vi "CTRE_Phoenix_MotorControl_GetAllConfigSettingsEnhanced.vi"(6 "timeoutMs":i32=50, 8 "error in (no error)":errorcluster, 11 "PhoenixMotorControlDevRef":T12={"DeviceStatus"={"status"=FALSE, "code"=0, "source"=""}, "Type"=enum."PWM", "PWM"={"PWM Channel"=enum."PWM 1", "DeadBand"={"Name"="", "maxPositivePwm"=0, "minPositivePwm"=0, "centerPwm"=0, "maxNegativePwm"=0, "minNegativePwm"=0, "angularRange"=0}}, "CAN"={"Device Number"=0, "SetOutput VI Ref"=variant(enum8{"Percent VBus", "Current", "Speed", "Position", "Voltage"} enum."Percent VBus"), "GetOutput VI Ref"=variant(refnum<k1> refnum), "Enable VI Ref"=variant(dbl 12.0), "Disable VI Ref"=variant(enum8{"Percent VBus", "Speed", "Position", "Slave", "Unchanged / Invalid", "Voltage Compensation", "Current", "Motion Profile"} enum."Percent VBus"), "Data"=variant}, "Invert"=FALSE, "DIO PWM"={"PWM \"Enable\" Channel"=enum."Invalid", "DIOChannel"=enum."Invalid", "PWM Rate"=0.0}}) -> (0 "error out":errorcluster, 2 "Enhanced Motor Controller Configurables":T1={"Base Configurables"={"openLoopRamp"=0.0, "closedLoopRamp"=0.0, "peakOutputForward"=1.0, "peakOutputReverse"=-1.0, "nominalOutputForward"=0.0, "nominalOutputReverse"=0.0, "neutralDeadband"=0.04, "voltageCompSaturation"=0.0, "voltageMeasurementFilter"=32, "velocityMeasurementPeriod"=100, "velocityMeasurementWindow"=64, "forwardSoftLimitThreshold"=64, "reverseSoftLimitThreshold"=64, "forwardSoftLimitEnable"=FALSE, "reverseSoftLimitEnable"=FALSE, "slot0"={"P"=0.0, "I"=0.0, "D"=0.0, "F"=0.0, "integralZone"=0.0, "allowableClosedLoopError"=0, "maxIntegralAccumulator"=0.0, "closedLoopPeakOutput"=1.0, "closedLoopPeriod"=1}, "slot1"={"P"=0.0, "I"=0.0, "D"=0.0, "F"=0.0, "integralZone"=0.0, "allowableClosedLoopError"=0, "maxIntegralAccumulator"=0.0, "closedLoopPeakOutput"=1.0, "closedLoopPeriod"=1}, "slot2"={"P"=0.0, "I"=0.0, "D"=0.0, "F"=0.0, "integralZone"=0.0, "allowableClosedLoopError"=0, "maxIntegralAccumulator"=0.0, "closedLoopPeakOutput"=1.0, "closedLoopPeriod"=1}, "slot3"={"P"=0.0, "I"=0.0, "D"=0.0, "F"=0.0, "integralZone"=0.0, "allowableClosedLoopError"=0, "maxIntegralAccumulator"=0.0, "closedLoopPeakOutput"=1.0, "closedLoopPeriod"=1}, "auxPIDPolarity"=FALSE, "remoteFilter0"={"remoteSensorDeviceID"=0, "remoteSensorSource"=enum."Off"}, "remoteFilter1"={"remoteSensorDeviceID"=0, "remoteSensorSource"=enum."Off"}, "motionCruiseVelocity"=0, "motionAcceleration"=0, "motionProfileTrajectoryPeriod"=0, "feedbackNotContinuous"=FALSE, "remoteSensorClosedLoopDisableNeutralOnLOS"=FALSE, "clearPositionOnLimitF"=FALSE, "clearPositionOnLimitR"=FALSE, "clearPositionOnQuadIdx"=FALSE, "limitSwitchDisableNeutralOnLOS"=FALSE, "softLimitDisableNeutralOnLOS"=FALSE, "pulseWidthPeriod_EdgesPerRot"=1, "pulseWidthPeriod_FilterWindowSz"=1, "customParam"={"customParam0"=0, "customParam1"=0}, "trajectoryInterpolationEnable"=TRUE}, "primaryPID"={"selectedFeedbackCoefficient"=1.0, "selectedFeedbackSensor"=0}, "auxiliaryPID"={"selectedFeedbackCoefficient"=1.0, "selectedFeedbackSensor"=0}, "sum0Term"=0, "sum1Term"=0, "diff0Term"=0, "diff1Term"=0, "forwardLimitSwitchNormal"=enum."Normally Open", "reverseLimitSwitchNormal"=enum."Normally Open", "forwardLimitSwitchDeviceID"=0, "reverseLimitSwitchDeviceID"=0, "forwardLimitSwitchSource"=enum."Feedback Connector", "reverseLimitSwitchSource"=enum."Feedback Connector", "peakCurrentLimit"=1, "peakCurrentDuration"=1, "continuousCurrentLimit"=1} {"diff1Term" items=["QuadEncoder"=0, "Analog"=2, "Tachometer"=4, "Pulse Width Encoded Position"=8, "Remote Source 0"=11, "Remote Source 1"=12, "Software Emulated"=15]; "diff0Term" items=["QuadEncoder"=0, "Analog"=2, "Tachometer"=4, "Pulse Width Encoded Position"=8, "Remote Source 0"=11, "Remote Source 1"=12, "Software Emulated"=15]; "sum1Term" items=["QuadEncoder"=0, "Analog"=2, "Tachometer"=4, "Pulse Width Encoded Position"=8, "Remote Source 0"=11, "Remote Source 1"=12, "Software Emulated"=15]; "sum0Term" items=["QuadEncoder"=0, "Analog"=2, "Tachometer"=4, "Pulse Width Encoded Position"=8, "Remote Source 0"=11, "Remote Source 1"=12, "Software Emulated"=15]; "auxiliaryPID"."selectedFeedbackSensor" items=["QuadEncoder"=0, "Analog"=2, "Tachometer"=4, "Pulse Width Encoded Position"=8, "Sensor Sum (S0 + S1)"=9, "Sensor Difference (D0 - D1)"=10, "Remote Source 0"=11, "Remote Source 1"=12, "Software Emulated"=15]; "primaryPID"."selectedFeedbackSensor" items=["QuadEncoder"=0, "Analog"=2, "Tachometer"=4, "Pulse Width Encoded Position"=8, "Sensor Sum (S0 + S1)"=9, "Sensor Difference (D0 - D1)"=10, "Remote Source 0"=11, "Remote Source 1"=12, "Software Emulated"=15]; "Base Configurables"."velocityMeasurementPeriod" items=["Period_1ms"=1, "Period_2ms"=2, "Period_5ms"=5, "Period_10ms"=10, "Period_20ms"=20, "Period_25ms"=25, "Period_50ms"=50, "Period_100ms"=100]}, 3 "PhoenixMotorControlDevRef":T12={"DeviceStatus"={"status"=FALSE, "code"=0, "source"=""}, "Type"=enum."PWM", "PWM"={"PWM Channel"=enum."PWM 1", "DeadBand"={"Name"="", "maxPositivePwm"=0, "minPositivePwm"=0, "centerPwm"=0, "maxNegativePwm"=0, "minNegativePwm"=0, "angularRange"=0}}, "CAN"={"Device Number"=0, "SetOutput VI Ref"=variant(enum8{"Percent VBus", "Current", "Speed", "Position", "Voltage"} enum."Percent VBus"), "GetOutput VI Ref"=variant(refnum<k1> refnum), "Enable VI Ref"=variant(dbl 12.0), "Disable VI Ref"=variant(enum8{"Percent VBus", "Speed", "Position", "Slave", "Unchanged / Invalid", "Voltage Compensation", "Current", "Motion Profile"} enum."Percent VBus"), "Data"=variant}, "Invert"=FALSE, "DIO PWM"={"PWM \"Enable\" Channel"=enum."Invalid", "DIOChannel"=enum."Invalid", "PWM Rate"=0.0}})   [LabVIEW 2020]
doc: "Gets all the slot persistant settings"
uses:
  <vilib>/Rock Robotics/WPI/MotorControl/WPI_MotorControlDeviceRef.ctl
  <vilib>/Rock Robotics/WPI/MotorControl/WPI_MotorControlType.ctl
  <vilib>/Rock Robotics/SystemInterfaces/DIO/FPGA_DIOPWMChannel.ctl
  <vilib>/Rock Robotics/WPI/PWM/WPI_PWMDeadband.ctl
  <vilib>/Rock Robotics/SystemInterfaces/DIO/FPGA_DIOChannel.ctl
  <vilib>/Rock Robotics/WPI/ThirdParty/Phoenix-LabVIEW/Motor Controller/Controls/CTRE_Phoenix_MotorControl_EnhancedMotorControllerConfigurables.ctl
  <vilib>/Rock Robotics/WPI/ThirdParty/Phoenix-LabVIEW/Motor Controller/Controls/CTRE_Phoenix_MotorControl_BaseConfigurables.ctl
  <vilib>/Rock Robotics/WPI/ThirdParty/Phoenix-LabVIEW/Motor Controller/Controls/CTRE_Phoenix_MotorControl_VelocityMeasurementPeriod.ctl
  <vilib>/Rock Robotics/WPI/ThirdParty/Phoenix-LabVIEW/Motor Controller/Controls/CTRE_Phoenix_MotorControl_SlotStructure.ctl
  <vilib>/Rock Robotics/WPI/ThirdParty/Phoenix-LabVIEW/Motor Controller/Controls/CTRE_Phoenix_MotorControl_FilterStruct.ctl
  <vilib>/Rock Robotics/WPI/ThirdParty/Phoenix-LabVIEW/Motor Controller/Controls/CTRE_Phoenix_MotorControl_RemoteSourceType.ctl
  <vilib>/Rock Robotics/WPI/ThirdParty/Phoenix-LabVIEW/Controls/CTRE_Phoenix_CustomParamConfiguration.ctl
  <vilib>/Rock Robotics/WPI/ThirdParty/Phoenix-LabVIEW/Motor Controller/Controls/CTRE_Phoenix_MotorControl_FeedbackDevice.ctl
  <vilib>/Rock Robotics/WPI/ThirdParty/Phoenix-LabVIEW/Motor Controller/Controls/CTRE_Phoenix_MotorControl_SensorTermFeedbackDevice_Enhanced.ctl
  <vilib>/Rock Robotics/WPI/ThirdParty/Phoenix-LabVIEW/Motor Controller/Controls/CTRE_Phoenix_MotorControl_LimitSwitchNormal.ctl
  <vilib>/Rock Robotics/WPI/ThirdParty/Phoenix-LabVIEW/Motor Controller/Controls/CTRE_Phoenix_MotorControl_LimitSwitchSource_Local.ctl
  <vilib>/Rock Robotics/WPI/ThirdParty/Phoenix-LabVIEW/Controls/CTRE_Phoenix_Params.ctl
panel:
  # "Sum and Diff terms are ways to select more than one sensor as a feedback device. \n Sum 0 is the first feedback device to be used for the Sum term.\n Sum 1 is the feedback device to be added to Sum 0 for the Sum term.\n Diff 0 and Diff 1 work in a similar manner."
  # "These are only applicable\nif using a remote limit switch.\n\nLocal limit switches/no limit\nswitches do not use this."
  # "Current is below Continuous threshold AND\n\n(Requested output is weaker** than applied motor\noutput OR is in the opposite direction).\n/\nMotor output is set to requested output."
  # "Current is above Peak* Threshold for Peak Duration.\n/\nReduce motor output (towards neutral)."
  # "Current is below Continuous threshold.\n/\nRamp motor output towards requested output."
  # "Current is above Continuous threshold.\n/\nReduce motor output (towards neutral)."
  # "Current Limiting is NOT enabled\nby default.\nCall this VI to enable."
  # "*If the configured Peak Threshold is less than the Continuous Threshold, the applied Peak Threshold is set equal to the Configured Continuous Threshold in firmware.\n** Both requested output and applied motor output are in the same direction, and requested output is closer to neutral."
  # "False: Primary Output = PID[0] + PID[1]  ---  Auxiliary Output = PID[0] - PID[1]\nTrue:  Primary Output = PID[0] - PID[1] --- Auxiliary Output = PID[0] + PID[1]"
  # "Enable the motion profile executor to perform linear interpolation between profile points.  Defaults to True."
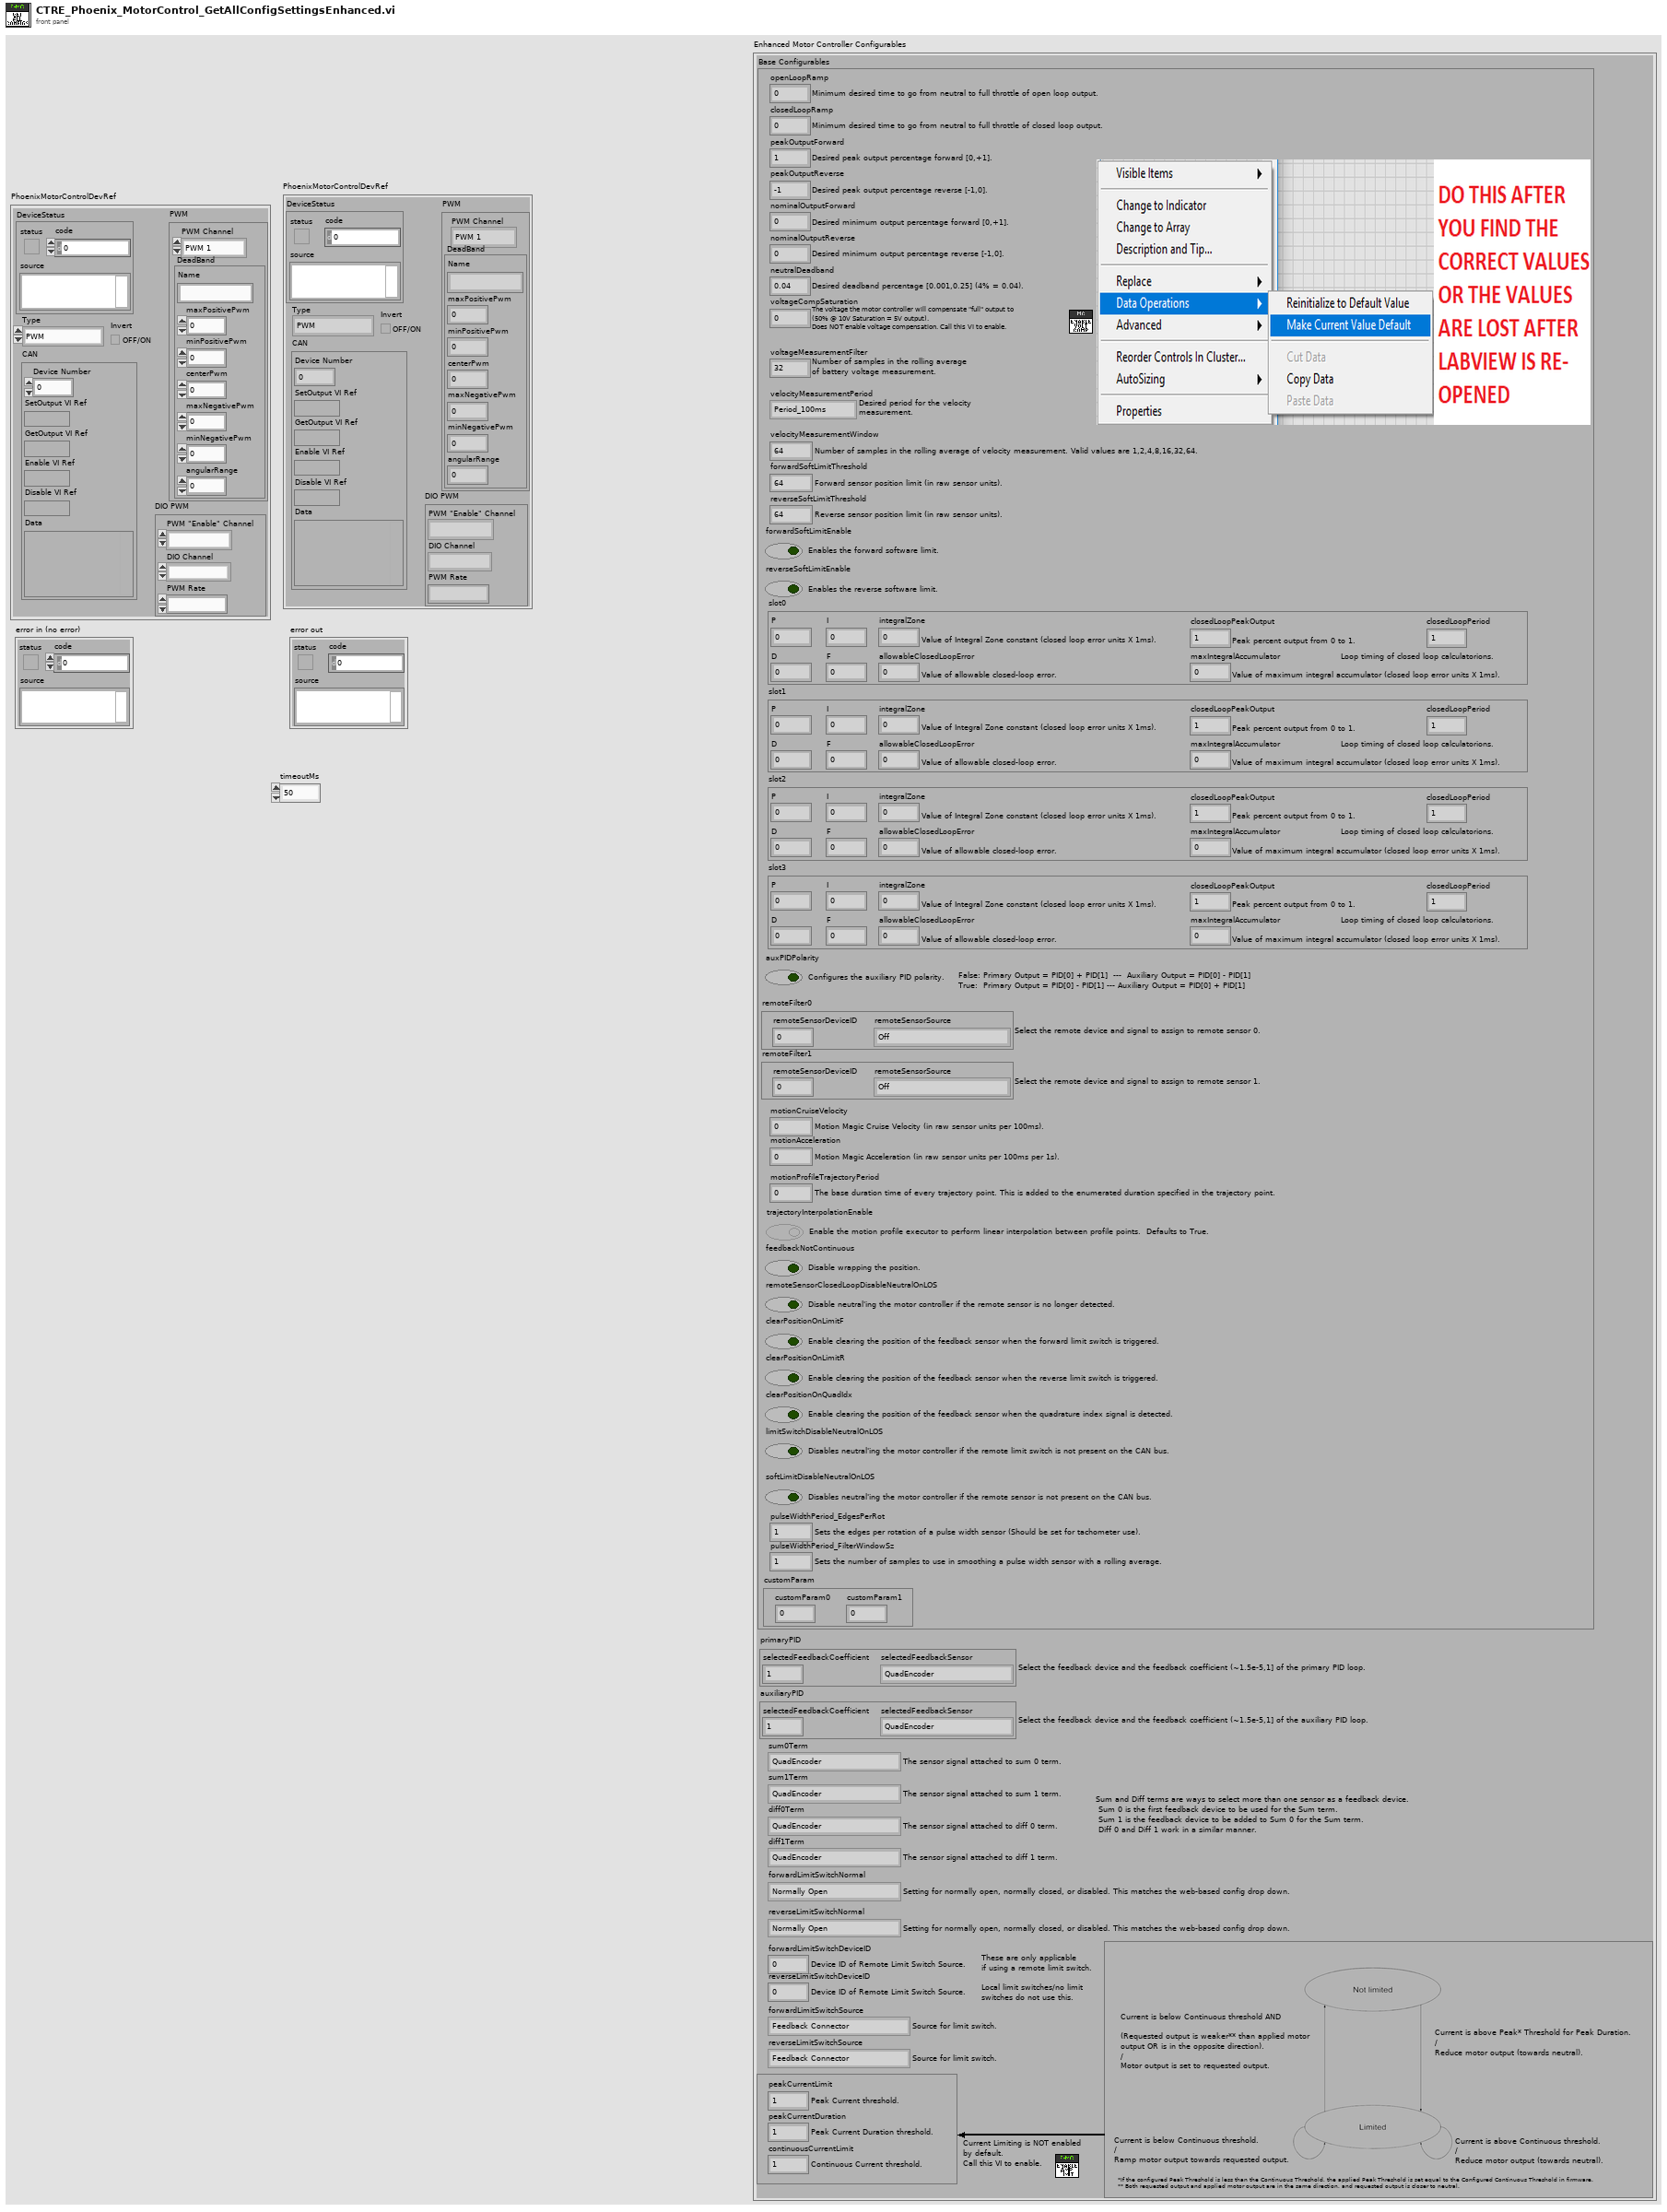
[diagram p1: front panel]
types:
  T1 = typedef "CTRE_Phoenix_MotorControl_EnhancedMotorControllerConfigurables.ctl" = cluster{"Base Configurables":T2, "primaryPID":cluster{"selectedFeedbackCoefficient":dbl, "selectedFeedbackSensor":T8}, "auxiliaryPID":cluster{"selectedFeedbackCoefficient":dbl, "selectedFeedbackSensor":T8}, "sum0Term":T9, "sum1Term":T9, "diff0Term":T9, "diff1Term":T9, "forwardLimitSwitchNormal":T10, "reverseLimitSwitchNormal":T10, "forwardLimitSwitchDeviceID":i32, "reverseLimitSwitchDeviceID":i32, "forwardLimitSwitchSource":T11, "reverseLimitSwitchSource":T11, "peakCurrentLimit":i32, "peakCurrentDuration":i32, "continuousCurrentLimit":i32}
  T2 = typedef "CTRE_Phoenix_MotorControl_BaseConfigurables.ctl" = cluster{"openLoopRamp":dbl, "closedLoopRamp":dbl, "peakOutputForward":dbl, "peakOutputReverse":dbl, "nominalOutputForward":dbl, "nominalOutputReverse":dbl, "neutralDeadband":dbl, "voltageCompSaturation":dbl, "voltageMeasurementFilter":i32, "velocityMeasurementPeriod":T3, "velocityMeasurementWindow":i32, "forwardSoftLimitThreshold":i32, "reverseSoftLimitThreshold":i32, "forwardSoftLimitEnable":bool, "reverseSoftLimitEnable":bool, "slot0":T4, "slot1":T4, "slot2":T4, "slot3":T4, "auxPIDPolarity":bool, "remoteFilter0":T5, "remoteFilter1":T5, "motionCruiseVelocity":i32, "motionAcceleration":i32, "motionProfileTrajectoryPeriod":i32, "feedbackNotContinuous":bool, "remoteSensorClosedLoopDisableNeutralOnLOS":bool, "clearPositionOnLimitF":bool, "clearPositionOnLimitR":bool, "clearPositionOnQuadIdx":bool, "limitSwitchDisableNeutralOnLOS":bool, "softLimitDisableNeutralOnLOS":bool, "pulseWidthPeriod_EdgesPerRot":i32, "pulseWidthPeriod_FilterWindowSz":i32, "customParam":T7, "trajectoryInterpolationEnable":bool}
  T3 = typedef "CTRE_Phoenix_MotorControl_VelocityMeasurementPeriod.ctl" = u16
  T4 = typedef "CTRE_Phoenix_MotorControl_SlotStructure.ctl" = cluster{"P":dbl, "I":dbl, "D":dbl, "F":dbl, "integralZone":dbl, "allowableClosedLoopError":i32, "maxIntegralAccumulator":dbl, "closedLoopPeakOutput":dbl, "closedLoopPeriod":i32}
  T5 = typedef "CTRE_Phoenix_MotorControl_FilterStruct.ctl" = cluster{"remoteSensorDeviceID":u8, "remoteSensorSource":T6}
  T6 = typedef "CTRE_Phoenix_MotorControl_RemoteSourceType.ctl" = enum16{"Off", "Talon SRX Selected Sensor", "Pigeon IMU Yaw", "Pigeon IMU Pitch", "Pigeon IMU Roll", "CANifier Quadrature", "CANifier PWM Input 0", "CANifier PWM Input 1", "CANifier PWM Input 2", "CANifier PWM Input 3", "Gadgeteer Pigeon Yaw", "Gadgeteer Pigeon Pitch", "Gadgeteer Pigeon Roll", "CANCoder"}
  T7 = typedef "CTRE_Phoenix_CustomParamConfiguration.ctl" = cluster{"customParam0":i32, "customParam1":i32}
  T8 = typedef "CTRE_Phoenix_MotorControl_FeedbackDevice.ctl" = i8
  T9 = typedef "CTRE_Phoenix_MotorControl_SensorTermFeedbackDevice_Enhanced.ctl" = i8
  T10 = typedef "CTRE_Phoenix_MotorControl_LimitSwitchNormal.ctl" = enum16{"Normally Open", "Normally Closed", "Disabled"}
  T11 = typedef "CTRE_Phoenix_MotorControl_LimitSwitchSource_Local.ctl" = enum16{"Feedback Connector", "Remote Talon SRX", "Remote CANifier", "Deactivated"}
  T12 = typedef "WPI_MotorControlDeviceRef.ctl" = cluster{"DeviceStatus":errorcluster, "Type":T13, "PWM":cluster{"PWM Channel":T14, "DeadBand":T15}, "CAN":cluster{"Device Number":u8, "SetOutput VI Ref":variant, "GetOutput VI Ref":variant, "Enable VI Ref":variant, "Disable VI Ref":variant, "Data":variant}, "Invert":bool, "DIO PWM":cluster{"PWM \"Enable\" Channel":T14, "DIOChannel":T16, "PWM Rate":dbl}}
  T13 = typedef "WPI_MotorControlType.ctl" = enum16{"PWM", "CAN", "DIO PWM"}
  T14 = typedef "FPGA_DIOPWMChannel.ctl" = enum8{"PWM 0", "PWM 1", "PWM 2", "PWM 3", "PWM 4", "PWM 5", "PWM 6", "PWM 7", "PWM 8", "PWM 9", "PWM MXP 0", "PWM MXP 1", "PWM MXP 2", "PWM MXP 3", "PWM MXP 4", "PWM MXP 5", "PWM MXP 6", "PWM MXP 7", "PWM MXP 8", "PWM MXP 9", "Invalid"}
  T15 = typedef "WPI_PWMDeadband.ctl" = cluster{"Name":string, "maxPositivePwm":i32, "minPositivePwm":i32, "centerPwm":i32, "maxNegativePwm":i32, "minNegativePwm":i32, "angularRange":u16}
  T16 = typedef "FPGA_DIOChannel.ctl" = enum8{"DIO 0", "DIO 1", "DIO 2", "DIO 3", "DIO 4", "DIO 5", "DIO 6", "DIO 7", "DIO 8", "DIO 9", "DIO MXP 0", "DIO MXP 1", "DIO MXP 2", "DIO MXP 3", "DIO MXP 4", "DIO MXP 5", "DIO MXP 6", "DIO MXP 7", "DIO MXP 8", "DIO MXP 9", "DIO MXP 10", "DIO MXP 11", "DIO MXP 12", "DIO MXP 13", "DIO MXP 14", "DIO MXP 15", "SPI Port CS1", "SPI Port CS2", "SPI Port CS3", "SPI Port MISO", "SPI Port MOSI", "Invalid"}
  T17 = typedef "CTRE_Phoenix_Params.ctl" = u16
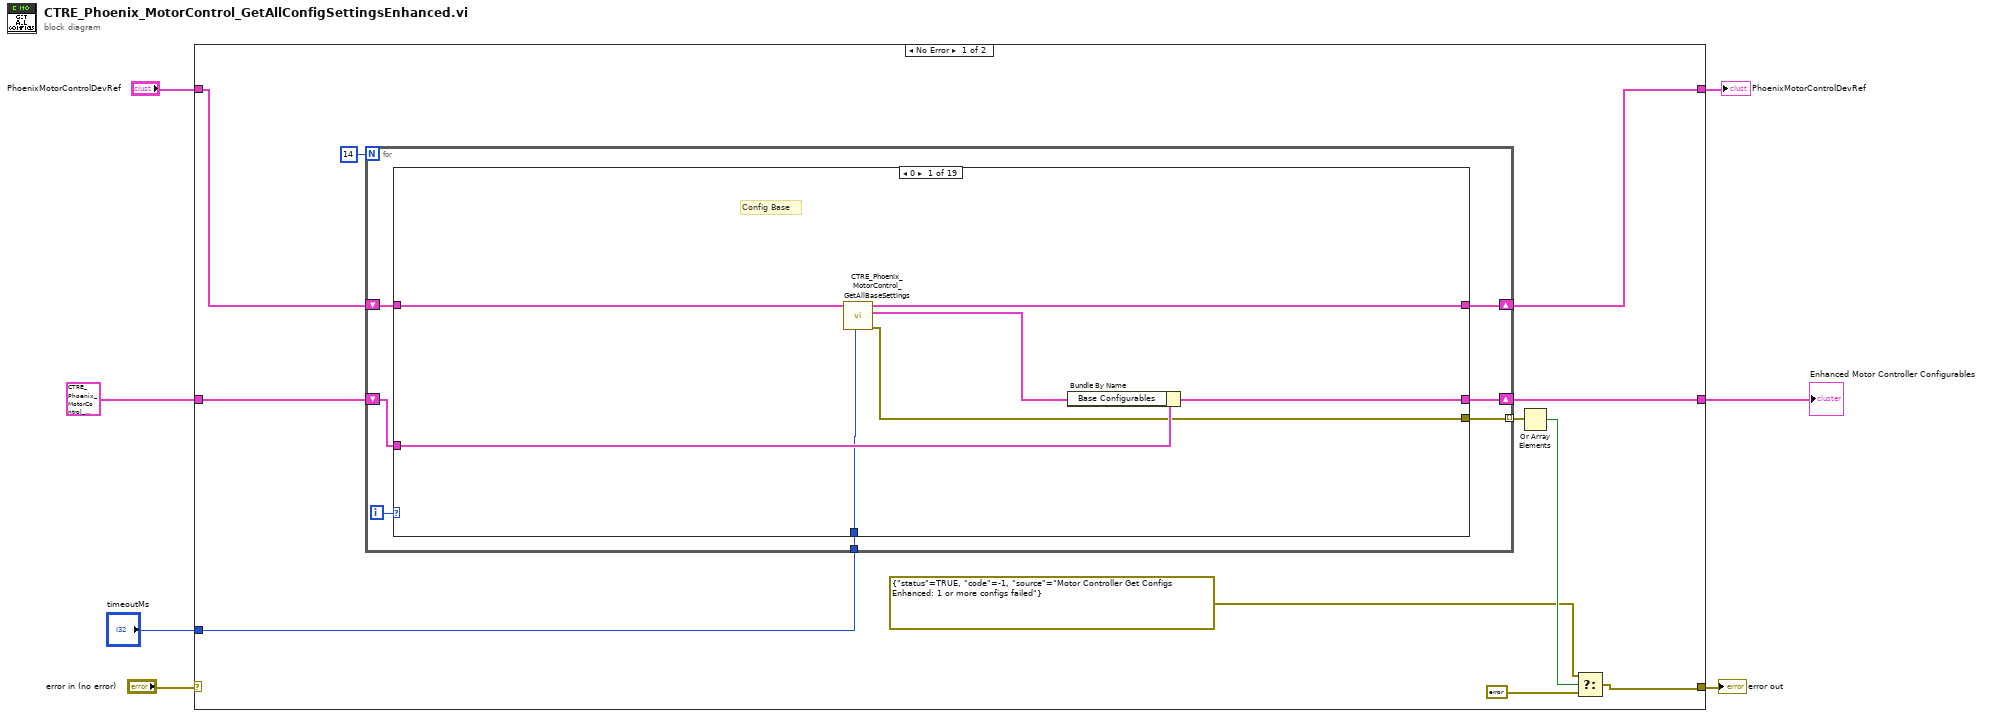
[diagram p0: block diagram]
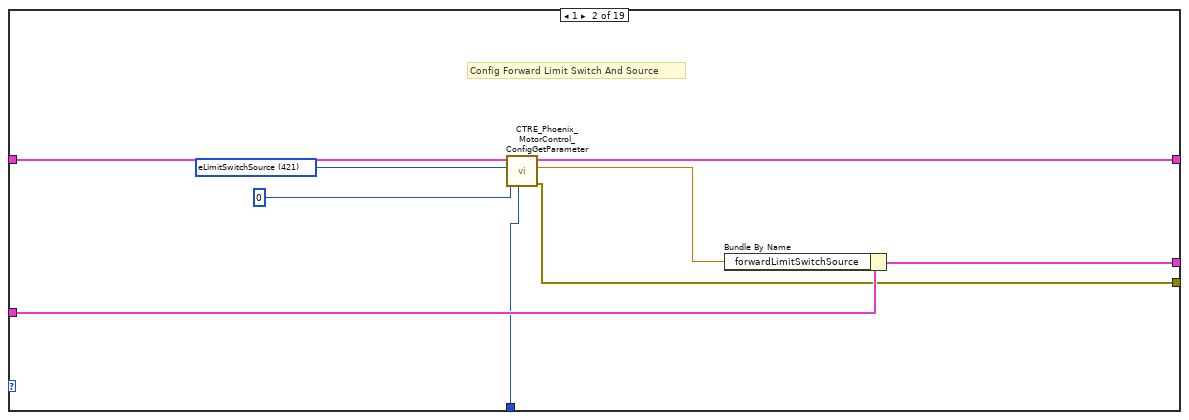
[diagram p2: hidden frame]
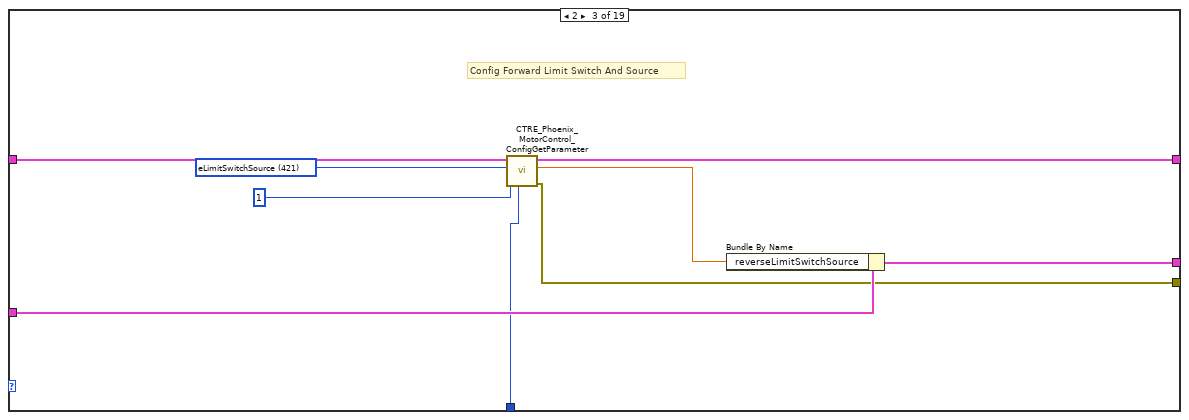
[diagram p3: hidden frame]
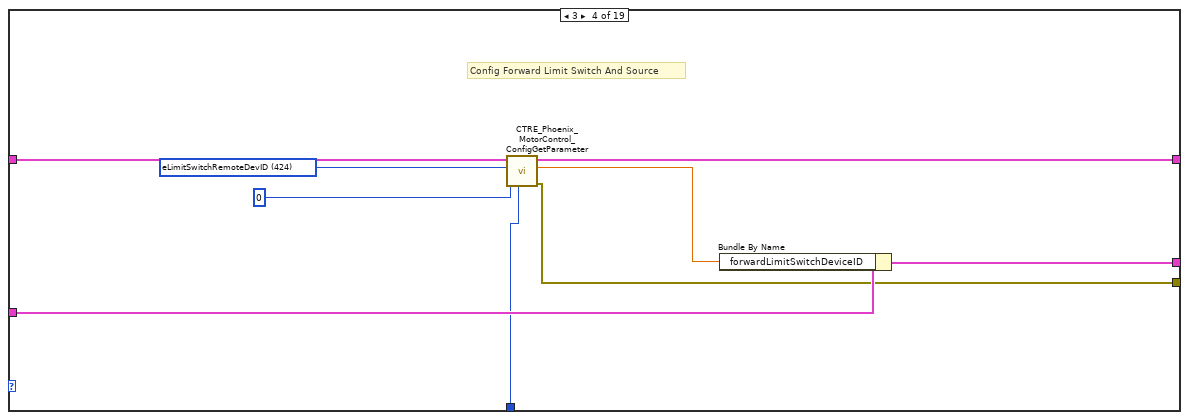
[diagram p4: hidden frame]
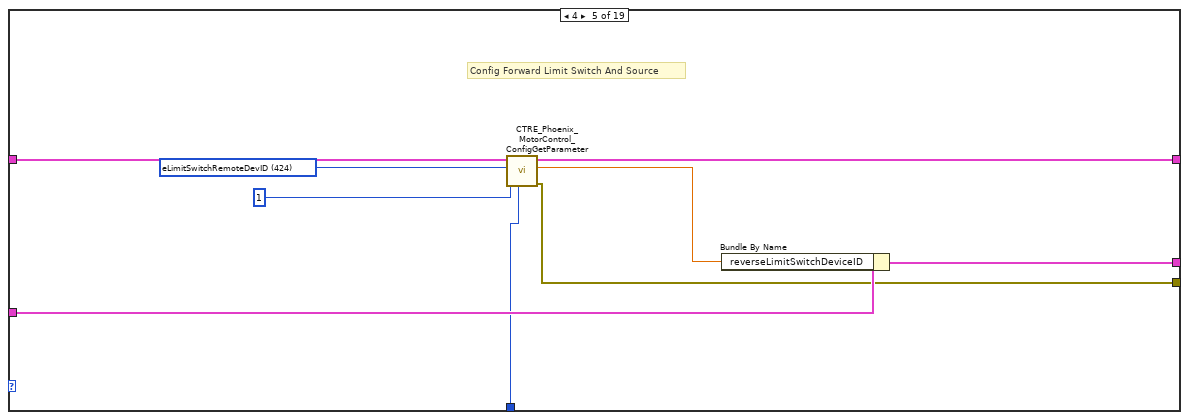
[diagram p5: hidden frame]
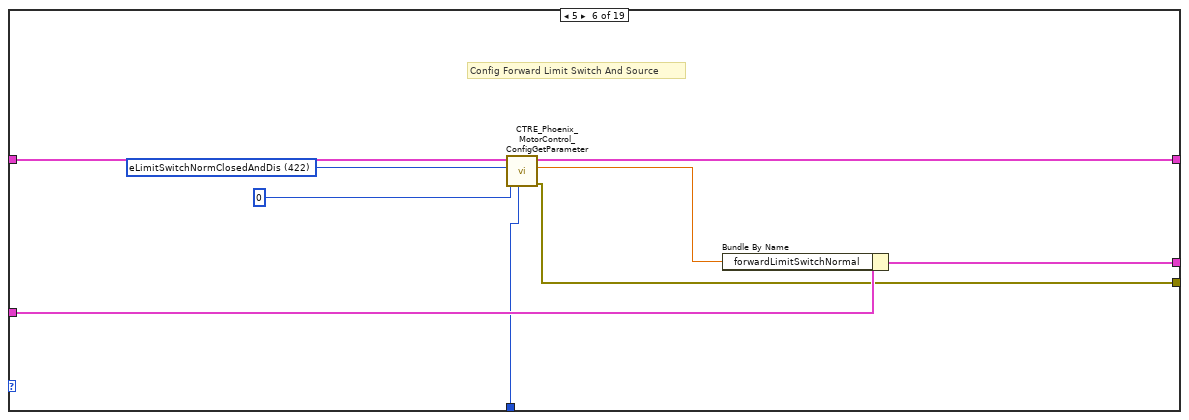
[diagram p6: hidden frame]
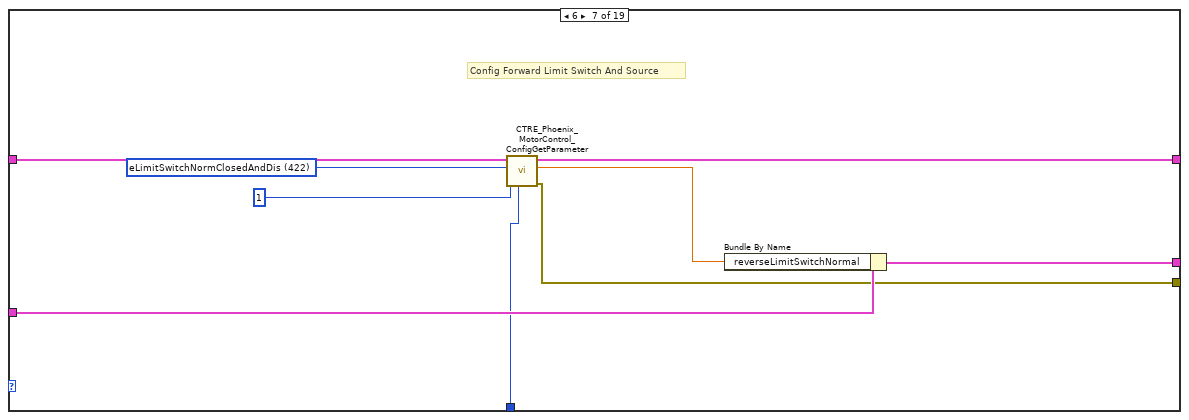
[diagram p7: hidden frame]
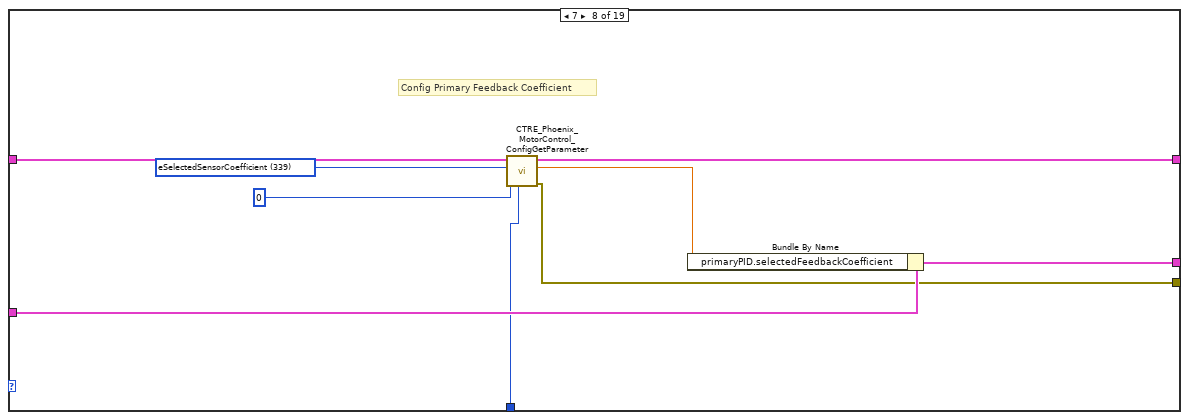
[diagram p8: hidden frame]
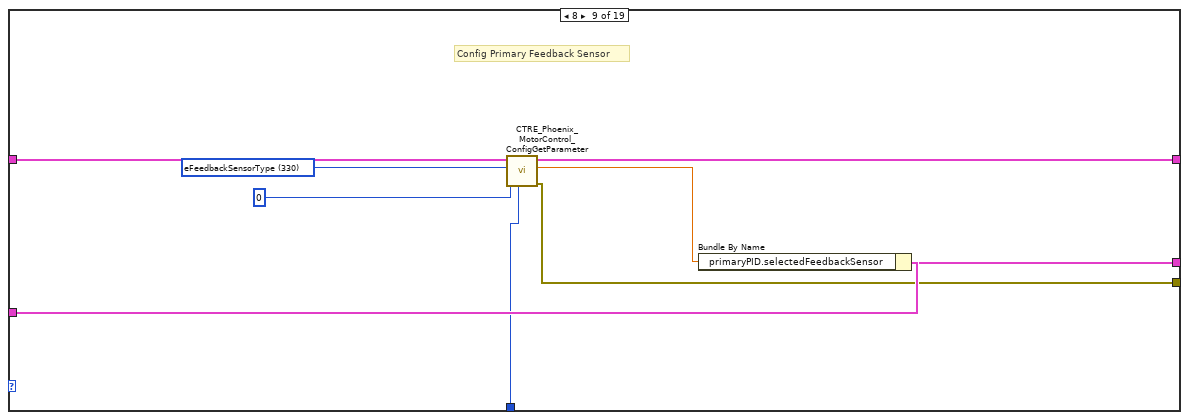
[diagram p9: hidden frame]
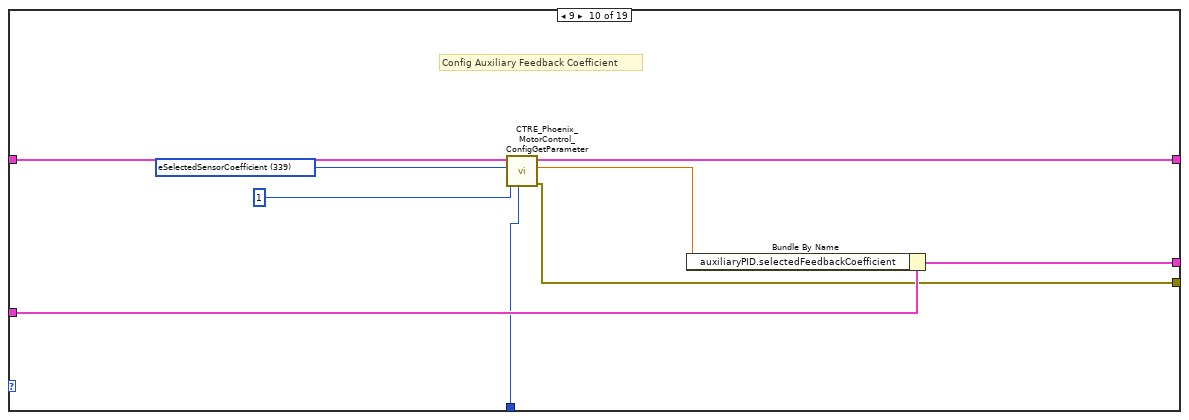
[diagram p10: hidden frame]
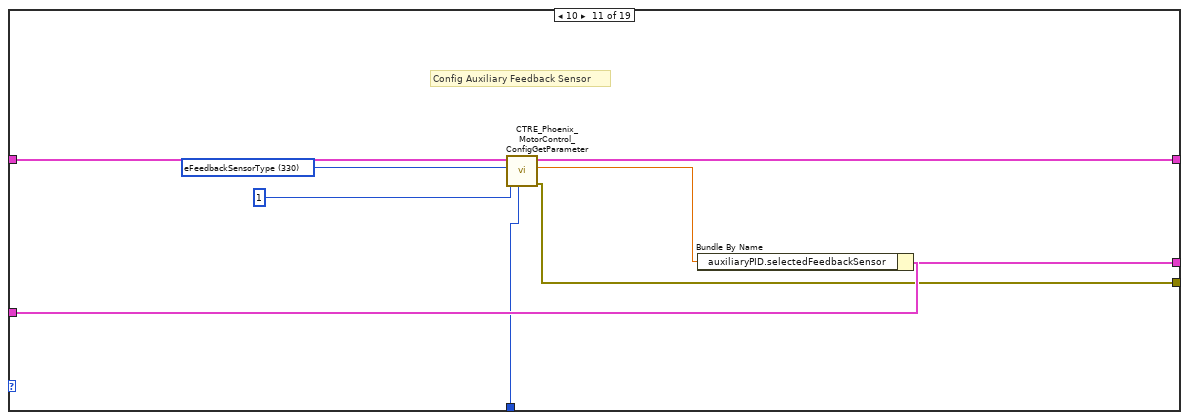
[diagram p11: hidden frame]
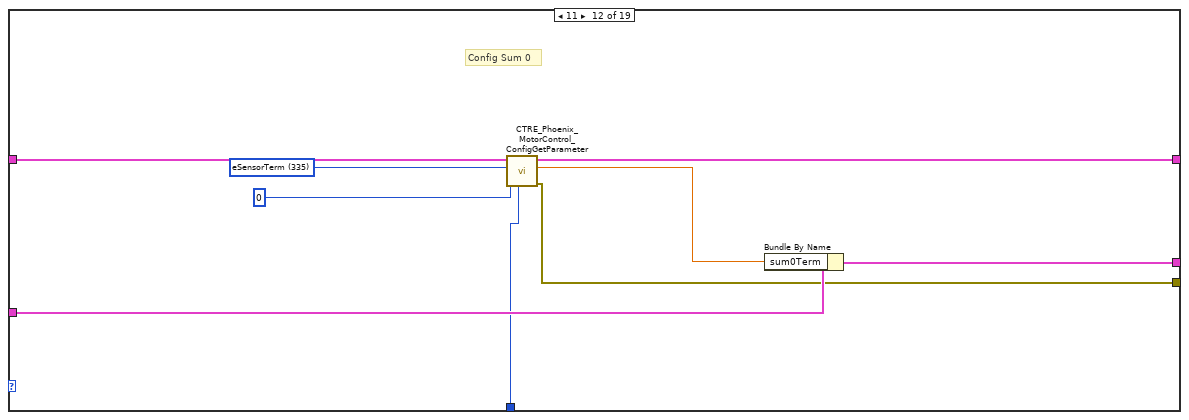
[diagram p12: hidden frame]
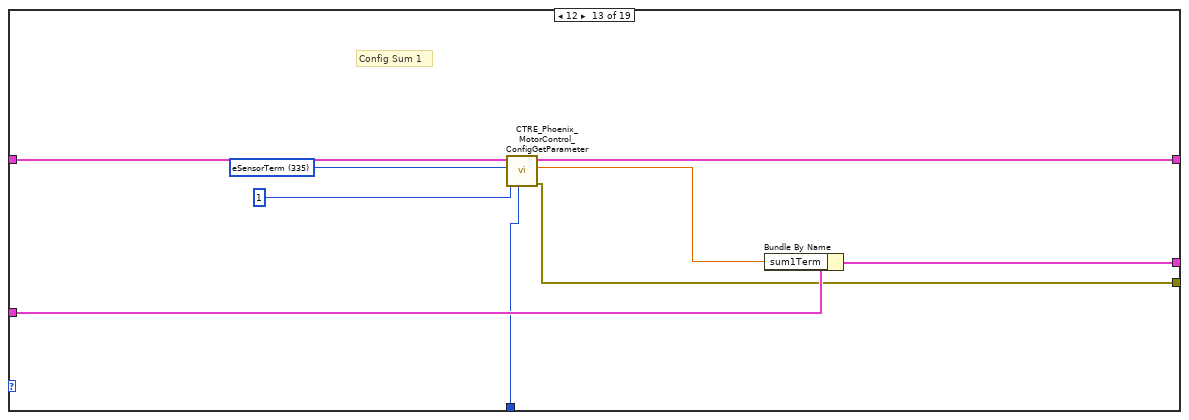
[diagram p13: hidden frame]
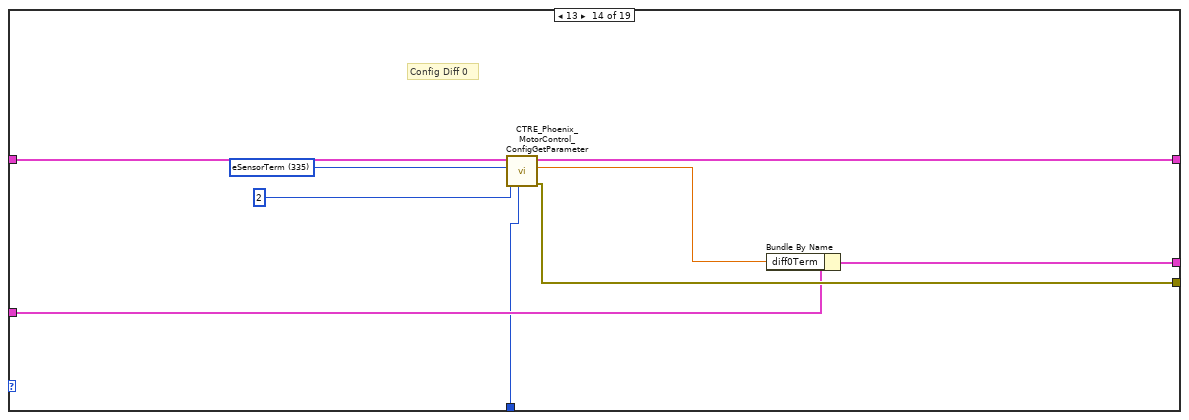
[diagram p14: hidden frame]
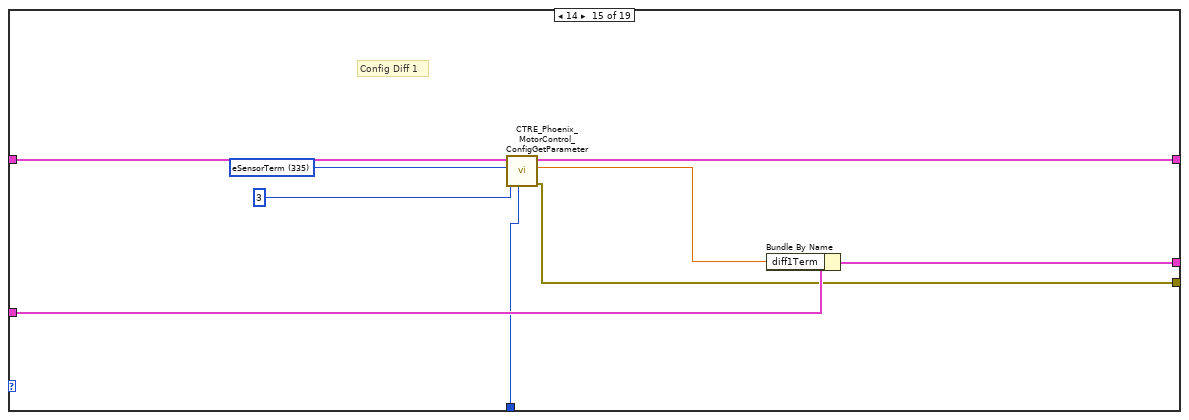
[diagram p15: hidden frame]
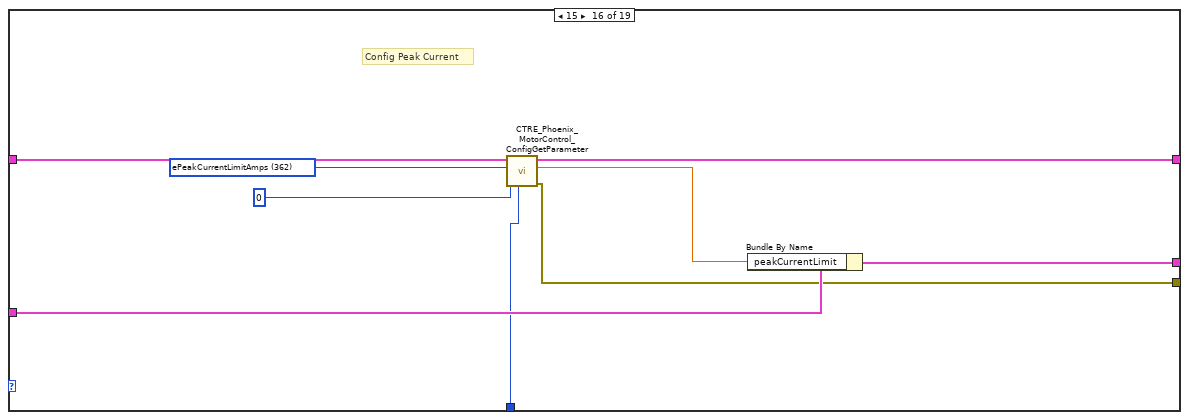
[diagram p16: hidden frame]
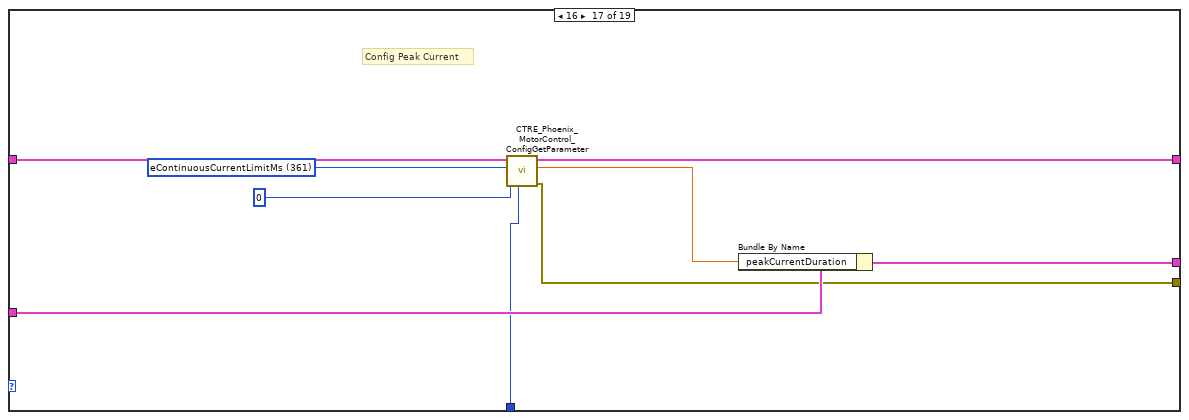
[diagram p17: hidden frame]
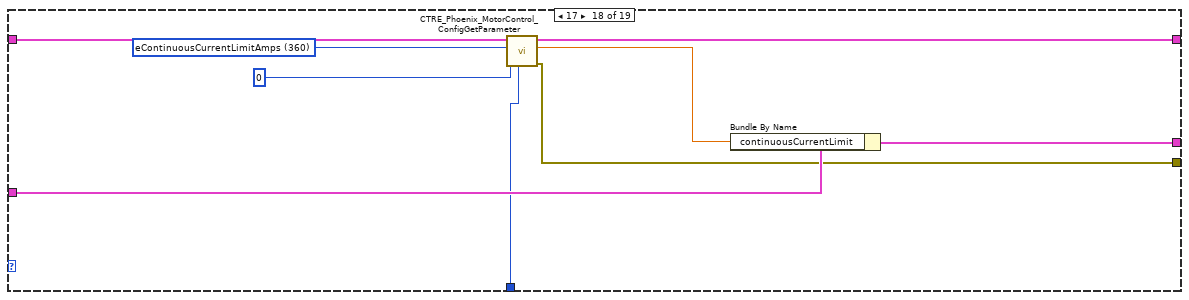
[diagram p18: hidden frame]
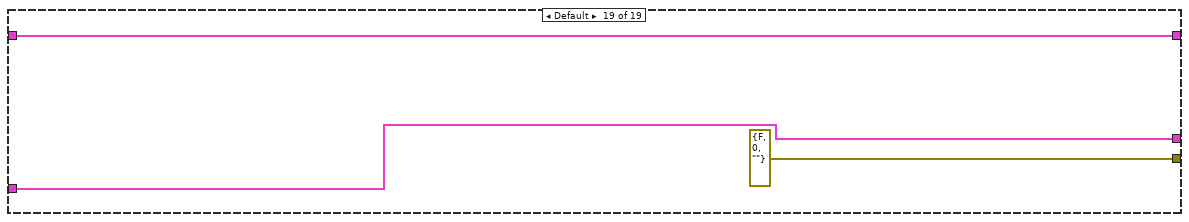
[diagram p19: hidden frame]
diagram:
  n1 = case shown="No Error" "error in (no error)" {
    selector: "error in (no error)" -> [_ w191]
    tunnel: [w15 w191] -> w7
    tunnel: "PhoenixMotorControlDevRef" -> [w18 w190]
    tunnel: [w17 w190] -> w5
    tunnel: "timeoutMs" -> [w16 _]
    tunnel: [w9 w189] -> w2
    tunnel: T1 {"Base Configurables"={"openLoopRamp"=0.0, "closedLoopRamp"=0.0, "peakOutputForward"=1.0, "peakOutputReverse"=-1.0, "nominalOutputForward"=0.0, "nominalOutputReverse"=0.0, "neutralDeadband"=0.04, "voltageCompSaturation"=0.0, "voltageMeasurementFilter"=32, "velocityMeasurementPeriod"=100, "velocityMeasurementWindow"=64, "forwardSoftLimitThreshold"=64, "reverseSoftLimitThreshold"=64, "forwardSoftLimitEnable"=FALSE, "reverseSoftLimitEnable"=FALSE, "slot0"={"P"=0.0, "I"=0.0, "D"=0.0, "F"=0.0, "integralZone"=0.0, "allowableClosedLoopError"=0, "maxIntegralAccumulator"=0.0, "closedLoopPeakOutput"=1.0, "closedLoopPeriod"=1}, "slot1"={"P"=0.0, "I"=0.0, "D"=0.0, "F"=0.0, "integralZone"=0.0, "allowableClosedLoopError"=0, "maxIntegralAccumulator"=0.0, "closedLoopPeakOutput"=1.0, "closedLoopPeriod"=1}, "slot2"={"P"=0.0, "I"=0.0, "D"=0.0, "F"=0.0, "integralZone"=0.0, "allowableClosedLoopError"=0, "maxIntegralAccumulator"=0.0, "closedLoopPeakOutput"=1.0, "closedLoopPeriod"=1}, "slot3"={"P"=0.0, "I"=0.0, "D"=0.0, "F"=0.0, "integralZone"=0.0, "allowableClosedLoopError"=0, "maxIntegralAccumulator"=0.0, "closedLoopPeakOutput"=1.0, "closedLoopPeriod"=1}, "auxPIDPolarity"=FALSE, "remoteFilter0"={"remoteSensorDeviceID"=0, "remoteSensorSource"=enum."Talon SRX Selected Sensor"}, "remoteFilter1"={"remoteSensorDeviceID"=0, "remoteSensorSource"=enum."Talon SRX Selected Sensor"}, "motionCruiseVelocity"=0, "motionAcceleration"=0, "motionProfileTrajectoryPeriod"=0, "feedbackNotContinuous"=FALSE, "remoteSensorClosedLoopDisableNeutralOnLOS"=FALSE, "clearPositionOnLimitF"=FALSE, "clearPositionOnLimitR"=FALSE, "clearPositionOnQuadIdx"=FALSE, "limitSwitchDisableNeutralOnLOS"=FALSE, "softLimitDisableNeutralOnLOS"=FALSE, "pulseWidthPeriod_EdgesPerRot"=1, "pulseWidthPeriod_FilterWindowSz"=1, "customParam"={"customParam0"=0, "customParam1"=0}, "trajectoryInterpolationEnable"=TRUE}, "primaryPID"={"selectedFeedbackCoefficient"=1.0, "selectedFeedbackSensor"=0}, "auxiliaryPID"={"selectedFeedbackCoefficient"=1.0, "selectedFeedbackSensor"=0}, "sum0Term"=0, "sum1Term"=0, "diff0Term"=0, "diff1Term"=0, "forwardLimitSwitchNormal"=enum."Normally Open", "reverseLimitSwitchNormal"=enum."Normally Open", "forwardLimitSwitchDeviceID"=0, "reverseLimitSwitchDeviceID"=0, "forwardLimitSwitchSource"=enum."Feedback Connector", "reverseLimitSwitchSource"=enum."Feedback Connector", "peakCurrentLimit"=1, "peakCurrentDuration"=1, "continuousCurrentLimit"=1} ("Enhanced Motor Controller Configurables 2") -> [w8 w189]
    frame No Error {
      n2 = for {
        N: 14 -> [_]
        tunnel: w16 -> [w23]
        shift-right: [w24] -> w17
        shift-left: w18 -> [w25]
        tunnel: [w21] -> w11 mode=indexing
        shift-right: [w19] -> w9
        shift-left: w8 -> [w20]
        i -> [w22]
        n3 = case shown="0" w22 {
          tunnel: w25 -> [w30 w38 w47 w56 w65 w74 w83 w91 w101 w109 w119 w128 w137 w142 w155 w164 w173 w182 w188]
          tunnel: [w29 w33 w42 w51 w60 w69 w78 w90 w96 w105 w114 w123 w132 w144 w150 w159 w168 w177 w188] -> w24
          tunnel: w23 -> [w27 w36 w45 w54 w63 w72 w81 w87 w99 w108 w117 w126 w135 w141 w153 w162 w171 w180 _]
          tunnel: [w26 w34 w43 w52 w61 w70 w79 w88 w98 w107 w116 w125 w134 w145 w151 w161 w170 w179 errorcluster {"status"=FALSE, "code"=0, "source"=""} ("error out")] -> w21
          tunnel: w20 -> [w32 w37 w46 w55 w64 w73 w82 w92 w100 w110 w118 w127 w136 w143 w154 w163 w172 w181 w186]
          tunnel: [w31 w35 w44 w53 w62 w71 w80 w89 w97 w106 w115 w124 w133 w146 w152 w160 w169 w178 w186] -> w19
          frame 0 {
            # "Config Base"
            n4 = call <vilib>:"CTRE_Phoenix_MotorControl_GetAllBaseSettings.vi"("timeoutMs"=w27, "PhoenixMotorControlDevRef"=w30) -> ("error out"=w26:errorcluster, "Base Configurables"=w28:T2, "PhoenixMotorControlDevRef"=w29:T12)  [unwired: 7 in]
            n5 = Bundle By Name(cluster=w32, "Base Configurables"=w28) -> (w31:T1)
          }
          frame 1 {
            w41 = T17 421 items=["eOnBoot_BrakeMode"=31, "eQuadFilterEn"=91, "eQuadIdxPolarity"=108, "eClearPositionOnIdx"=100, "eMotionProfileHasUnderrunErr"=119, "eMotionProfileTrajectoryPointDurationMs"=120, "eClearPosOnLimitF"=144, "eClearPosOnLimitR"=145, "eStatusFramePeriod"=300, "eOpenLoopRamp"=301, "eClosedLoopRamp"=302, "eNeutralDeadband"=303, "ePeakPosOutput"=305, "eNominalPosOutput"=306, "ePeakNegOutput"=307, "eNominalNegOutput"=308, "eProfileParamSlot_P"=310, "eProfileParamSlot_I"=311, "eProfileParamSlot_D"=312, "eProfileParamSlot_F"=313, "eProfileParamSlot_IZone"=314, "eProfileParamSlot_AllowableErr"=315, "eProfileParamSlot_MaxIAccum"=316, "eProfileParamSlot_PeakOutput"=317, "eClearPositionOnLimitF"=320, "eClearPositionOnLimitR"=321, "eClearPositionOnQuadIdx"=322, "eSampleVelocityPeriod"=325, "eSampleVelocityWindow"=326, "eFeedbackSensorType"=330, "eSelectedSensorPosition"=331, "eFeedbackNotContinuous"=332, "eRemoteSensorSource"=333, "eRemoteSensorDeviceID"=334, "eSensorTerm"=335, "eRemoteSensorClosedLoopDisableNeutralOnLOS"=336, "ePIDLoopPolarity"=337, "ePIDLoopPeriod"=338, "eSelectedSensorCoefficient"=339, "eForwardSoftLimitThreshold"=340, "eReverseSoftLimitThreshold"=341, "eForwardSoftLimitEnable"=342, "eReverseSoftLimitEnable"=343, "eNominalBatteryVoltage"=350, "eBatterVoltageFilterSize"=351, "eContinuousCurrentLimitAmps"=360, "eContinuousCurrentLimitMs"=361, "ePeakCurrentLimitAmps"=362, "eClosedLoopIAccum"=370, "eCustomParam"=380, "eStickyFaults"=390, "eAnalogPosition"=400, "eQuadraturePosition"=401, "ePulseWidthPosition"=402, "eMotMag_Accel"=410, "eMotMag_VelCruise"=411, "eLimitSwitchSource"=421, "eLimitSwitchNormClosedAndDis"=422, "eLimitSwitchDisabledNeutralOnLOS"=423, "eLimitSwitchRemoteDevID"=424, "eSoftLimitDisabledNeutralOnLOS"=425] ("Parameter")
            # "Config Forward Limit Switch And Source"
            n6 = call <vilib>:"CTRE_Phoenix_MotorControl_ConfigGetParameter.vi"("timeoutMs"=w36, "ordinal"=0, "Parameter"=w41, "PhoenixMotorControlDevRef"=w38) -> ("error out"=w34:errorcluster, "value"=w39:dbl, "PhoenixMotorControlDevRef"=w33:T12)  [unwired: 5 in]
            n7 = Bundle By Name(cluster=w37, "forwardLimitSwitchSource"=w39) -> (w35:T1)
          }
          frame 2 {
            w50 = T17 421 items=["eOnBoot_BrakeMode"=31, "eQuadFilterEn"=91, "eQuadIdxPolarity"=108, "eClearPositionOnIdx"=100, "eMotionProfileHasUnderrunErr"=119, "eMotionProfileTrajectoryPointDurationMs"=120, "eClearPosOnLimitF"=144, "eClearPosOnLimitR"=145, "eStatusFramePeriod"=300, "eOpenLoopRamp"=301, "eClosedLoopRamp"=302, "eNeutralDeadband"=303, "ePeakPosOutput"=305, "eNominalPosOutput"=306, "ePeakNegOutput"=307, "eNominalNegOutput"=308, "eProfileParamSlot_P"=310, "eProfileParamSlot_I"=311, "eProfileParamSlot_D"=312, "eProfileParamSlot_F"=313, "eProfileParamSlot_IZone"=314, "eProfileParamSlot_AllowableErr"=315, "eProfileParamSlot_MaxIAccum"=316, "eProfileParamSlot_PeakOutput"=317, "eClearPositionOnLimitF"=320, "eClearPositionOnLimitR"=321, "eClearPositionOnQuadIdx"=322, "eSampleVelocityPeriod"=325, "eSampleVelocityWindow"=326, "eFeedbackSensorType"=330, "eSelectedSensorPosition"=331, "eFeedbackNotContinuous"=332, "eRemoteSensorSource"=333, "eRemoteSensorDeviceID"=334, "eSensorTerm"=335, "eRemoteSensorClosedLoopDisableNeutralOnLOS"=336, "ePIDLoopPolarity"=337, "ePIDLoopPeriod"=338, "eSelectedSensorCoefficient"=339, "eForwardSoftLimitThreshold"=340, "eReverseSoftLimitThreshold"=341, "eForwardSoftLimitEnable"=342, "eReverseSoftLimitEnable"=343, "eNominalBatteryVoltage"=350, "eBatterVoltageFilterSize"=351, "eContinuousCurrentLimitAmps"=360, "eContinuousCurrentLimitMs"=361, "ePeakCurrentLimitAmps"=362, "eClosedLoopIAccum"=370, "eCustomParam"=380, "eStickyFaults"=390, "eAnalogPosition"=400, "eQuadraturePosition"=401, "ePulseWidthPosition"=402, "eMotMag_Accel"=410, "eMotMag_VelCruise"=411, "eLimitSwitchSource"=421, "eLimitSwitchNormClosedAndDis"=422, "eLimitSwitchDisabledNeutralOnLOS"=423, "eLimitSwitchRemoteDevID"=424, "eSoftLimitDisabledNeutralOnLOS"=425] ("Parameter")
            # "Config Forward Limit Switch And Source"
            n8 = call <vilib>:"CTRE_Phoenix_MotorControl_ConfigGetParameter.vi"("timeoutMs"=w45, "ordinal"=1, "Parameter"=w50, "PhoenixMotorControlDevRef"=w47) -> ("error out"=w43:errorcluster, "value"=w48:dbl, "PhoenixMotorControlDevRef"=w42:T12)  [unwired: 5 in]
            n9 = Bundle By Name(cluster=w46, "reverseLimitSwitchSource"=w48) -> (w44:T1)
          }
          frame 3 {
            w59 = T17 424 items=["eOnBoot_BrakeMode"=31, "eQuadFilterEn"=91, "eQuadIdxPolarity"=108, "eClearPositionOnIdx"=100, "eMotionProfileHasUnderrunErr"=119, "eMotionProfileTrajectoryPointDurationMs"=120, "eClearPosOnLimitF"=144, "eClearPosOnLimitR"=145, "eStatusFramePeriod"=300, "eOpenLoopRamp"=301, "eClosedLoopRamp"=302, "eNeutralDeadband"=303, "ePeakPosOutput"=305, "eNominalPosOutput"=306, "ePeakNegOutput"=307, "eNominalNegOutput"=308, "eProfileParamSlot_P"=310, "eProfileParamSlot_I"=311, "eProfileParamSlot_D"=312, "eProfileParamSlot_F"=313, "eProfileParamSlot_IZone"=314, "eProfileParamSlot_AllowableErr"=315, "eProfileParamSlot_MaxIAccum"=316, "eProfileParamSlot_PeakOutput"=317, "eClearPositionOnLimitF"=320, "eClearPositionOnLimitR"=321, "eClearPositionOnQuadIdx"=322, "eSampleVelocityPeriod"=325, "eSampleVelocityWindow"=326, "eFeedbackSensorType"=330, "eSelectedSensorPosition"=331, "eFeedbackNotContinuous"=332, "eRemoteSensorSource"=333, "eRemoteSensorDeviceID"=334, "eSensorTerm"=335, "eRemoteSensorClosedLoopDisableNeutralOnLOS"=336, "ePIDLoopPolarity"=337, "ePIDLoopPeriod"=338, "eSelectedSensorCoefficient"=339, "eForwardSoftLimitThreshold"=340, "eReverseSoftLimitThreshold"=341, "eForwardSoftLimitEnable"=342, "eReverseSoftLimitEnable"=343, "eNominalBatteryVoltage"=350, "eBatterVoltageFilterSize"=351, "eContinuousCurrentLimitAmps"=360, "eContinuousCurrentLimitMs"=361, "ePeakCurrentLimitAmps"=362, "eClosedLoopIAccum"=370, "eCustomParam"=380, "eStickyFaults"=390, "eAnalogPosition"=400, "eQuadraturePosition"=401, "ePulseWidthPosition"=402, "eMotMag_Accel"=410, "eMotMag_VelCruise"=411, "eLimitSwitchSource"=421, "eLimitSwitchNormClosedAndDis"=422, "eLimitSwitchDisabledNeutralOnLOS"=423, "eLimitSwitchRemoteDevID"=424, "eSoftLimitDisabledNeutralOnLOS"=425] ("Parameter")
            # "Config Forward Limit Switch And Source"
            n10 = call <vilib>:"CTRE_Phoenix_MotorControl_ConfigGetParameter.vi"("timeoutMs"=w54, "ordinal"=0, "Parameter"=w59, "PhoenixMotorControlDevRef"=w56) -> ("error out"=w52:errorcluster, "value"=w57:dbl, "PhoenixMotorControlDevRef"=w51:T12)  [unwired: 5 in]
            n11 = Bundle By Name(cluster=w55, "forwardLimitSwitchDeviceID"=w57) -> (w53:T1)
          }
          frame 4 {
            w68 = T17 424 items=["eOnBoot_BrakeMode"=31, "eQuadFilterEn"=91, "eQuadIdxPolarity"=108, "eClearPositionOnIdx"=100, "eMotionProfileHasUnderrunErr"=119, "eMotionProfileTrajectoryPointDurationMs"=120, "eClearPosOnLimitF"=144, "eClearPosOnLimitR"=145, "eStatusFramePeriod"=300, "eOpenLoopRamp"=301, "eClosedLoopRamp"=302, "eNeutralDeadband"=303, "ePeakPosOutput"=305, "eNominalPosOutput"=306, "ePeakNegOutput"=307, "eNominalNegOutput"=308, "eProfileParamSlot_P"=310, "eProfileParamSlot_I"=311, "eProfileParamSlot_D"=312, "eProfileParamSlot_F"=313, "eProfileParamSlot_IZone"=314, "eProfileParamSlot_AllowableErr"=315, "eProfileParamSlot_MaxIAccum"=316, "eProfileParamSlot_PeakOutput"=317, "eClearPositionOnLimitF"=320, "eClearPositionOnLimitR"=321, "eClearPositionOnQuadIdx"=322, "eSampleVelocityPeriod"=325, "eSampleVelocityWindow"=326, "eFeedbackSensorType"=330, "eSelectedSensorPosition"=331, "eFeedbackNotContinuous"=332, "eRemoteSensorSource"=333, "eRemoteSensorDeviceID"=334, "eSensorTerm"=335, "eRemoteSensorClosedLoopDisableNeutralOnLOS"=336, "ePIDLoopPolarity"=337, "ePIDLoopPeriod"=338, "eSelectedSensorCoefficient"=339, "eForwardSoftLimitThreshold"=340, "eReverseSoftLimitThreshold"=341, "eForwardSoftLimitEnable"=342, "eReverseSoftLimitEnable"=343, "eNominalBatteryVoltage"=350, "eBatterVoltageFilterSize"=351, "eContinuousCurrentLimitAmps"=360, "eContinuousCurrentLimitMs"=361, "ePeakCurrentLimitAmps"=362, "eClosedLoopIAccum"=370, "eCustomParam"=380, "eStickyFaults"=390, "eAnalogPosition"=400, "eQuadraturePosition"=401, "ePulseWidthPosition"=402, "eMotMag_Accel"=410, "eMotMag_VelCruise"=411, "eLimitSwitchSource"=421, "eLimitSwitchNormClosedAndDis"=422, "eLimitSwitchDisabledNeutralOnLOS"=423, "eLimitSwitchRemoteDevID"=424, "eSoftLimitDisabledNeutralOnLOS"=425] ("Parameter")
            # "Config Forward Limit Switch And Source"
            n12 = call <vilib>:"CTRE_Phoenix_MotorControl_ConfigGetParameter.vi"("timeoutMs"=w63, "ordinal"=1, "Parameter"=w68, "PhoenixMotorControlDevRef"=w65) -> ("error out"=w61:errorcluster, "value"=w66:dbl, "PhoenixMotorControlDevRef"=w60:T12)  [unwired: 5 in]
            n13 = Bundle By Name(cluster=w64, "reverseLimitSwitchDeviceID"=w66) -> (w62:T1)
          }
          frame 5 {
            w77 = T17 422 items=["eOnBoot_BrakeMode"=31, "eQuadFilterEn"=91, "eQuadIdxPolarity"=108, "eClearPositionOnIdx"=100, "eMotionProfileHasUnderrunErr"=119, "eMotionProfileTrajectoryPointDurationMs"=120, "eClearPosOnLimitF"=144, "eClearPosOnLimitR"=145, "eStatusFramePeriod"=300, "eOpenLoopRamp"=301, "eClosedLoopRamp"=302, "eNeutralDeadband"=303, "ePeakPosOutput"=305, "eNominalPosOutput"=306, "ePeakNegOutput"=307, "eNominalNegOutput"=308, "eProfileParamSlot_P"=310, "eProfileParamSlot_I"=311, "eProfileParamSlot_D"=312, "eProfileParamSlot_F"=313, "eProfileParamSlot_IZone"=314, "eProfileParamSlot_AllowableErr"=315, "eProfileParamSlot_MaxIAccum"=316, "eProfileParamSlot_PeakOutput"=317, "eClearPositionOnLimitF"=320, "eClearPositionOnLimitR"=321, "eClearPositionOnQuadIdx"=322, "eSampleVelocityPeriod"=325, "eSampleVelocityWindow"=326, "eFeedbackSensorType"=330, "eSelectedSensorPosition"=331, "eFeedbackNotContinuous"=332, "eRemoteSensorSource"=333, "eRemoteSensorDeviceID"=334, "eSensorTerm"=335, "eRemoteSensorClosedLoopDisableNeutralOnLOS"=336, "ePIDLoopPolarity"=337, "ePIDLoopPeriod"=338, "eSelectedSensorCoefficient"=339, "eForwardSoftLimitThreshold"=340, "eReverseSoftLimitThreshold"=341, "eForwardSoftLimitEnable"=342, "eReverseSoftLimitEnable"=343, "eNominalBatteryVoltage"=350, "eBatterVoltageFilterSize"=351, "eContinuousCurrentLimitAmps"=360, "eContinuousCurrentLimitMs"=361, "ePeakCurrentLimitAmps"=362, "eClosedLoopIAccum"=370, "eCustomParam"=380, "eStickyFaults"=390, "eAnalogPosition"=400, "eQuadraturePosition"=401, "ePulseWidthPosition"=402, "eMotMag_Accel"=410, "eMotMag_VelCruise"=411, "eLimitSwitchSource"=421, "eLimitSwitchNormClosedAndDis"=422, "eLimitSwitchDisabledNeutralOnLOS"=423, "eLimitSwitchRemoteDevID"=424, "eSoftLimitDisabledNeutralOnLOS"=425] ("Parameter")
            # "Config Forward Limit Switch And Source"
            n14 = call <vilib>:"CTRE_Phoenix_MotorControl_ConfigGetParameter.vi"("timeoutMs"=w72, "ordinal"=0, "Parameter"=w77, "PhoenixMotorControlDevRef"=w74) -> ("error out"=w70:errorcluster, "value"=w75:dbl, "PhoenixMotorControlDevRef"=w69:T12)  [unwired: 5 in]
            n15 = Bundle By Name(cluster=w73, "forwardLimitSwitchNormal"=w75) -> (w71:T1)
          }
          frame 6 {
            w86 = T17 422 items=["eOnBoot_BrakeMode"=31, "eQuadFilterEn"=91, "eQuadIdxPolarity"=108, "eClearPositionOnIdx"=100, "eMotionProfileHasUnderrunErr"=119, "eMotionProfileTrajectoryPointDurationMs"=120, "eClearPosOnLimitF"=144, "eClearPosOnLimitR"=145, "eStatusFramePeriod"=300, "eOpenLoopRamp"=301, "eClosedLoopRamp"=302, "eNeutralDeadband"=303, "ePeakPosOutput"=305, "eNominalPosOutput"=306, "ePeakNegOutput"=307, "eNominalNegOutput"=308, "eProfileParamSlot_P"=310, "eProfileParamSlot_I"=311, "eProfileParamSlot_D"=312, "eProfileParamSlot_F"=313, "eProfileParamSlot_IZone"=314, "eProfileParamSlot_AllowableErr"=315, "eProfileParamSlot_MaxIAccum"=316, "eProfileParamSlot_PeakOutput"=317, "eClearPositionOnLimitF"=320, "eClearPositionOnLimitR"=321, "eClearPositionOnQuadIdx"=322, "eSampleVelocityPeriod"=325, "eSampleVelocityWindow"=326, "eFeedbackSensorType"=330, "eSelectedSensorPosition"=331, "eFeedbackNotContinuous"=332, "eRemoteSensorSource"=333, "eRemoteSensorDeviceID"=334, "eSensorTerm"=335, "eRemoteSensorClosedLoopDisableNeutralOnLOS"=336, "ePIDLoopPolarity"=337, "ePIDLoopPeriod"=338, "eSelectedSensorCoefficient"=339, "eForwardSoftLimitThreshold"=340, "eReverseSoftLimitThreshold"=341, "eForwardSoftLimitEnable"=342, "eReverseSoftLimitEnable"=343, "eNominalBatteryVoltage"=350, "eBatterVoltageFilterSize"=351, "eContinuousCurrentLimitAmps"=360, "eContinuousCurrentLimitMs"=361, "ePeakCurrentLimitAmps"=362, "eClosedLoopIAccum"=370, "eCustomParam"=380, "eStickyFaults"=390, "eAnalogPosition"=400, "eQuadraturePosition"=401, "ePulseWidthPosition"=402, "eMotMag_Accel"=410, "eMotMag_VelCruise"=411, "eLimitSwitchSource"=421, "eLimitSwitchNormClosedAndDis"=422, "eLimitSwitchDisabledNeutralOnLOS"=423, "eLimitSwitchRemoteDevID"=424, "eSoftLimitDisabledNeutralOnLOS"=425] ("Parameter")
            # "Config Forward Limit Switch And Source"
            n16 = call <vilib>:"CTRE_Phoenix_MotorControl_ConfigGetParameter.vi"("timeoutMs"=w81, "ordinal"=1, "Parameter"=w86, "PhoenixMotorControlDevRef"=w83) -> ("error out"=w79:errorcluster, "value"=w84:dbl, "PhoenixMotorControlDevRef"=w78:T12)  [unwired: 5 in]
            n17 = Bundle By Name(cluster=w82, "reverseLimitSwitchNormal"=w84) -> (w80:T1)
          }
          frame 7 {
            w95 = T17 339 items=["eOnBoot_BrakeMode"=31, "eQuadFilterEn"=91, "eQuadIdxPolarity"=108, "eClearPositionOnIdx"=100, "eMotionProfileHasUnderrunErr"=119, "eMotionProfileTrajectoryPointDurationMs"=120, "eClearPosOnLimitF"=144, "eClearPosOnLimitR"=145, "eStatusFramePeriod"=300, "eOpenLoopRamp"=301, "eClosedLoopRamp"=302, "eNeutralDeadband"=303, "ePeakPosOutput"=305, "eNominalPosOutput"=306, "ePeakNegOutput"=307, "eNominalNegOutput"=308, "eProfileParamSlot_P"=310, "eProfileParamSlot_I"=311, "eProfileParamSlot_D"=312, "eProfileParamSlot_F"=313, "eProfileParamSlot_IZone"=314, "eProfileParamSlot_AllowableErr"=315, "eProfileParamSlot_MaxIAccum"=316, "eProfileParamSlot_PeakOutput"=317, "eClearPositionOnLimitF"=320, "eClearPositionOnLimitR"=321, "eClearPositionOnQuadIdx"=322, "eSampleVelocityPeriod"=325, "eSampleVelocityWindow"=326, "eFeedbackSensorType"=330, "eSelectedSensorPosition"=331, "eFeedbackNotContinuous"=332, "eRemoteSensorSource"=333, "eRemoteSensorDeviceID"=334, "eSensorTerm"=335, "eRemoteSensorClosedLoopDisableNeutralOnLOS"=336, "ePIDLoopPolarity"=337, "ePIDLoopPeriod"=338, "eSelectedSensorCoefficient"=339, "eForwardSoftLimitThreshold"=340, "eReverseSoftLimitThreshold"=341, "eForwardSoftLimitEnable"=342, "eReverseSoftLimitEnable"=343, "eNominalBatteryVoltage"=350, "eBatterVoltageFilterSize"=351, "eContinuousCurrentLimitAmps"=360, "eContinuousCurrentLimitMs"=361, "ePeakCurrentLimitAmps"=362, "eClosedLoopIAccum"=370, "eCustomParam"=380, "eStickyFaults"=390, "eAnalogPosition"=400, "eQuadraturePosition"=401, "ePulseWidthPosition"=402, "eMotMag_Accel"=410, "eMotMag_VelCruise"=411, "eLimitSwitchSource"=421, "eLimitSwitchNormClosedAndDis"=422, "eLimitSwitchDisabledNeutralOnLOS"=423, "eLimitSwitchRemoteDevID"=424, "eSoftLimitDisabledNeutralOnLOS"=425, "ePulseWidthPeriod_EdgesPerRot"=430, "ePulseWidthPeriod_FilterWindowSz"=431] ("Parameter")
            # "Config Primary Feedback Coefficient"
            n18 = call <vilib>:"CTRE_Phoenix_MotorControl_ConfigGetParameter.vi"("timeoutMs"=w87, "ordinal"=0, "Parameter"=w95, "PhoenixMotorControlDevRef"=w91) -> ("error out"=w88:errorcluster, "value"=w93:dbl, "PhoenixMotorControlDevRef"=w90:T12)  [unwired: 5 in]
            n19 = Bundle By Name(cluster=w92, "primaryPID.selectedFeedbackCoefficient"=w93) -> (w89:T1)
          }
          frame 8 {
            w104 = T17 330 items=["eOnBoot_BrakeMode"=31, "eQuadFilterEn"=91, "eQuadIdxPolarity"=108, "eClearPositionOnIdx"=100, "eMotionProfileHasUnderrunErr"=119, "eMotionProfileTrajectoryPointDurationMs"=120, "eClearPosOnLimitF"=144, "eClearPosOnLimitR"=145, "eStatusFramePeriod"=300, "eOpenLoopRamp"=301, "eClosedLoopRamp"=302, "eNeutralDeadband"=303, "ePeakPosOutput"=305, "eNominalPosOutput"=306, "ePeakNegOutput"=307, "eNominalNegOutput"=308, "eProfileParamSlot_P"=310, "eProfileParamSlot_I"=311, "eProfileParamSlot_D"=312, "eProfileParamSlot_F"=313, "eProfileParamSlot_IZone"=314, "eProfileParamSlot_AllowableErr"=315, "eProfileParamSlot_MaxIAccum"=316, "eProfileParamSlot_PeakOutput"=317, "eClearPositionOnLimitF"=320, "eClearPositionOnLimitR"=321, "eClearPositionOnQuadIdx"=322, "eSampleVelocityPeriod"=325, "eSampleVelocityWindow"=326, "eFeedbackSensorType"=330, "eSelectedSensorPosition"=331, "eFeedbackNotContinuous"=332, "eRemoteSensorSource"=333, "eRemoteSensorDeviceID"=334, "eSensorTerm"=335, "eRemoteSensorClosedLoopDisableNeutralOnLOS"=336, "ePIDLoopPolarity"=337, "ePIDLoopPeriod"=338, "eSelectedSensorCoefficient"=339, "eForwardSoftLimitThreshold"=340, "eReverseSoftLimitThreshold"=341, "eForwardSoftLimitEnable"=342, "eReverseSoftLimitEnable"=343, "eNominalBatteryVoltage"=350, "eBatterVoltageFilterSize"=351, "eContinuousCurrentLimitAmps"=360, "eContinuousCurrentLimitMs"=361, "ePeakCurrentLimitAmps"=362, "eClosedLoopIAccum"=370, "eCustomParam"=380, "eStickyFaults"=390, "eAnalogPosition"=400, "eQuadraturePosition"=401, "ePulseWidthPosition"=402, "eMotMag_Accel"=410, "eMotMag_VelCruise"=411, "eLimitSwitchSource"=421, "eLimitSwitchNormClosedAndDis"=422, "eLimitSwitchDisabledNeutralOnLOS"=423, "eLimitSwitchRemoteDevID"=424, "eSoftLimitDisabledNeutralOnLOS"=425, "ePulseWidthPeriod_EdgesPerRot"=430, "ePulseWidthPeriod_FilterWindowSz"=431] ("Parameter")
            # "Config Primary Feedback Sensor"
            n20 = call <vilib>:"CTRE_Phoenix_MotorControl_ConfigGetParameter.vi"("timeoutMs"=w99, "ordinal"=0, "Parameter"=w104, "PhoenixMotorControlDevRef"=w101) -> ("error out"=w98:errorcluster, "value"=w102:dbl, "PhoenixMotorControlDevRef"=w96:T12)  [unwired: 5 in]
            n21 = Bundle By Name(cluster=w100, "primaryPID.selectedFeedbackSensor"=w102) -> (w97:T1)
          }
          frame 9 {
            w113 = T17 339 items=["eOnBoot_BrakeMode"=31, "eQuadFilterEn"=91, "eQuadIdxPolarity"=108, "eClearPositionOnIdx"=100, "eMotionProfileHasUnderrunErr"=119, "eMotionProfileTrajectoryPointDurationMs"=120, "eClearPosOnLimitF"=144, "eClearPosOnLimitR"=145, "eStatusFramePeriod"=300, "eOpenLoopRamp"=301, "eClosedLoopRamp"=302, "eNeutralDeadband"=303, "ePeakPosOutput"=305, "eNominalPosOutput"=306, "ePeakNegOutput"=307, "eNominalNegOutput"=308, "eProfileParamSlot_P"=310, "eProfileParamSlot_I"=311, "eProfileParamSlot_D"=312, "eProfileParamSlot_F"=313, "eProfileParamSlot_IZone"=314, "eProfileParamSlot_AllowableErr"=315, "eProfileParamSlot_MaxIAccum"=316, "eProfileParamSlot_PeakOutput"=317, "eClearPositionOnLimitF"=320, "eClearPositionOnLimitR"=321, "eClearPositionOnQuadIdx"=322, "eSampleVelocityPeriod"=325, "eSampleVelocityWindow"=326, "eFeedbackSensorType"=330, "eSelectedSensorPosition"=331, "eFeedbackNotContinuous"=332, "eRemoteSensorSource"=333, "eRemoteSensorDeviceID"=334, "eSensorTerm"=335, "eRemoteSensorClosedLoopDisableNeutralOnLOS"=336, "ePIDLoopPolarity"=337, "ePIDLoopPeriod"=338, "eSelectedSensorCoefficient"=339, "eForwardSoftLimitThreshold"=340, "eReverseSoftLimitThreshold"=341, "eForwardSoftLimitEnable"=342, "eReverseSoftLimitEnable"=343, "eNominalBatteryVoltage"=350, "eBatterVoltageFilterSize"=351, "eContinuousCurrentLimitAmps"=360, "eContinuousCurrentLimitMs"=361, "ePeakCurrentLimitAmps"=362, "eClosedLoopIAccum"=370, "eCustomParam"=380, "eStickyFaults"=390, "eAnalogPosition"=400, "eQuadraturePosition"=401, "ePulseWidthPosition"=402, "eMotMag_Accel"=410, "eMotMag_VelCruise"=411, "eLimitSwitchSource"=421, "eLimitSwitchNormClosedAndDis"=422, "eLimitSwitchDisabledNeutralOnLOS"=423, "eLimitSwitchRemoteDevID"=424, "eSoftLimitDisabledNeutralOnLOS"=425, "ePulseWidthPeriod_EdgesPerRot"=430, "ePulseWidthPeriod_FilterWindowSz"=431] ("Parameter")
            # "Config Auxiliary Feedback Coefficient"
            n22 = call <vilib>:"CTRE_Phoenix_MotorControl_ConfigGetParameter.vi"("timeoutMs"=w108, "ordinal"=1, "Parameter"=w113, "PhoenixMotorControlDevRef"=w109) -> ("error out"=w107:errorcluster, "value"=w111:dbl, "PhoenixMotorControlDevRef"=w105:T12)  [unwired: 5 in]
            n23 = Bundle By Name(cluster=w110, "auxiliaryPID.selectedFeedbackCoefficient"=w111) -> (w106:T1)
          }
          frame 10 {
            w122 = T17 330 items=["eOnBoot_BrakeMode"=31, "eQuadFilterEn"=91, "eQuadIdxPolarity"=108, "eClearPositionOnIdx"=100, "eMotionProfileHasUnderrunErr"=119, "eMotionProfileTrajectoryPointDurationMs"=120, "eClearPosOnLimitF"=144, "eClearPosOnLimitR"=145, "eStatusFramePeriod"=300, "eOpenLoopRamp"=301, "eClosedLoopRamp"=302, "eNeutralDeadband"=303, "ePeakPosOutput"=305, "eNominalPosOutput"=306, "ePeakNegOutput"=307, "eNominalNegOutput"=308, "eProfileParamSlot_P"=310, "eProfileParamSlot_I"=311, "eProfileParamSlot_D"=312, "eProfileParamSlot_F"=313, "eProfileParamSlot_IZone"=314, "eProfileParamSlot_AllowableErr"=315, "eProfileParamSlot_MaxIAccum"=316, "eProfileParamSlot_PeakOutput"=317, "eClearPositionOnLimitF"=320, "eClearPositionOnLimitR"=321, "eClearPositionOnQuadIdx"=322, "eSampleVelocityPeriod"=325, "eSampleVelocityWindow"=326, "eFeedbackSensorType"=330, "eSelectedSensorPosition"=331, "eFeedbackNotContinuous"=332, "eRemoteSensorSource"=333, "eRemoteSensorDeviceID"=334, "eSensorTerm"=335, "eRemoteSensorClosedLoopDisableNeutralOnLOS"=336, "ePIDLoopPolarity"=337, "ePIDLoopPeriod"=338, "eSelectedSensorCoefficient"=339, "eForwardSoftLimitThreshold"=340, "eReverseSoftLimitThreshold"=341, "eForwardSoftLimitEnable"=342, "eReverseSoftLimitEnable"=343, "eNominalBatteryVoltage"=350, "eBatterVoltageFilterSize"=351, "eContinuousCurrentLimitAmps"=360, "eContinuousCurrentLimitMs"=361, "ePeakCurrentLimitAmps"=362, "eClosedLoopIAccum"=370, "eCustomParam"=380, "eStickyFaults"=390, "eAnalogPosition"=400, "eQuadraturePosition"=401, "ePulseWidthPosition"=402, "eMotMag_Accel"=410, "eMotMag_VelCruise"=411, "eLimitSwitchSource"=421, "eLimitSwitchNormClosedAndDis"=422, "eLimitSwitchDisabledNeutralOnLOS"=423, "eLimitSwitchRemoteDevID"=424, "eSoftLimitDisabledNeutralOnLOS"=425, "ePulseWidthPeriod_EdgesPerRot"=430, "ePulseWidthPeriod_FilterWindowSz"=431] ("Parameter")
            # "Config Auxiliary Feedback Sensor"
            n24 = call <vilib>:"CTRE_Phoenix_MotorControl_ConfigGetParameter.vi"("timeoutMs"=w117, "ordinal"=1, "Parameter"=w122, "PhoenixMotorControlDevRef"=w119) -> ("error out"=w116:errorcluster, "value"=w120:dbl, "PhoenixMotorControlDevRef"=w114:T12)  [unwired: 5 in]
            n25 = Bundle By Name(cluster=w118, "auxiliaryPID.selectedFeedbackSensor"=w120) -> (w115:T1)
          }
          frame 11 {
            w131 = T17 335 items=["eOnBoot_BrakeMode"=31, "eQuadFilterEn"=91, "eQuadIdxPolarity"=108, "eClearPositionOnIdx"=100, "eMotionProfileHasUnderrunErr"=119, "eMotionProfileTrajectoryPointDurationMs"=120, "eClearPosOnLimitF"=144, "eClearPosOnLimitR"=145, "eStatusFramePeriod"=300, "eOpenLoopRamp"=301, "eClosedLoopRamp"=302, "eNeutralDeadband"=303, "ePeakPosOutput"=305, "eNominalPosOutput"=306, "ePeakNegOutput"=307, "eNominalNegOutput"=308, "eProfileParamSlot_P"=310, "eProfileParamSlot_I"=311, "eProfileParamSlot_D"=312, "eProfileParamSlot_F"=313, "eProfileParamSlot_IZone"=314, "eProfileParamSlot_AllowableErr"=315, "eProfileParamSlot_MaxIAccum"=316, "eProfileParamSlot_PeakOutput"=317, "eClearPositionOnLimitF"=320, "eClearPositionOnLimitR"=321, "eClearPositionOnQuadIdx"=322, "eSampleVelocityPeriod"=325, "eSampleVelocityWindow"=326, "eFeedbackSensorType"=330, "eSelectedSensorPosition"=331, "eFeedbackNotContinuous"=332, "eRemoteSensorSource"=333, "eRemoteSensorDeviceID"=334, "eSensorTerm"=335, "eRemoteSensorClosedLoopDisableNeutralOnLOS"=336, "ePIDLoopPolarity"=337, "ePIDLoopPeriod"=338, "eSelectedSensorCoefficient"=339, "eForwardSoftLimitThreshold"=340, "eReverseSoftLimitThreshold"=341, "eForwardSoftLimitEnable"=342, "eReverseSoftLimitEnable"=343, "eNominalBatteryVoltage"=350, "eBatterVoltageFilterSize"=351, "eContinuousCurrentLimitAmps"=360, "eContinuousCurrentLimitMs"=361, "ePeakCurrentLimitAmps"=362, "eClosedLoopIAccum"=370, "eCustomParam"=380, "eStickyFaults"=390, "eAnalogPosition"=400, "eQuadraturePosition"=401, "ePulseWidthPosition"=402, "eMotMag_Accel"=410, "eMotMag_VelCruise"=411, "eLimitSwitchSource"=421, "eLimitSwitchNormClosedAndDis"=422, "eLimitSwitchDisabledNeutralOnLOS"=423, "eLimitSwitchRemoteDevID"=424, "eSoftLimitDisabledNeutralOnLOS"=425, "ePulseWidthPeriod_EdgesPerRot"=430, "ePulseWidthPeriod_FilterWindowSz"=431] ("Parameter")
            # "Config Sum 0"
            n26 = call <vilib>:"CTRE_Phoenix_MotorControl_ConfigGetParameter.vi"("timeoutMs"=w126, "ordinal"=0, "Parameter"=w131, "PhoenixMotorControlDevRef"=w128) -> ("error out"=w125:errorcluster, "value"=w129:dbl, "PhoenixMotorControlDevRef"=w123:T12)  [unwired: 5 in]
            n27 = Bundle By Name(cluster=w127, "sum0Term"=w129) -> (w124:T1)
          }
          frame 12 {
            w140 = T17 335 items=["eOnBoot_BrakeMode"=31, "eQuadFilterEn"=91, "eQuadIdxPolarity"=108, "eClearPositionOnIdx"=100, "eMotionProfileHasUnderrunErr"=119, "eMotionProfileTrajectoryPointDurationMs"=120, "eClearPosOnLimitF"=144, "eClearPosOnLimitR"=145, "eStatusFramePeriod"=300, "eOpenLoopRamp"=301, "eClosedLoopRamp"=302, "eNeutralDeadband"=303, "ePeakPosOutput"=305, "eNominalPosOutput"=306, "ePeakNegOutput"=307, "eNominalNegOutput"=308, "eProfileParamSlot_P"=310, "eProfileParamSlot_I"=311, "eProfileParamSlot_D"=312, "eProfileParamSlot_F"=313, "eProfileParamSlot_IZone"=314, "eProfileParamSlot_AllowableErr"=315, "eProfileParamSlot_MaxIAccum"=316, "eProfileParamSlot_PeakOutput"=317, "eClearPositionOnLimitF"=320, "eClearPositionOnLimitR"=321, "eClearPositionOnQuadIdx"=322, "eSampleVelocityPeriod"=325, "eSampleVelocityWindow"=326, "eFeedbackSensorType"=330, "eSelectedSensorPosition"=331, "eFeedbackNotContinuous"=332, "eRemoteSensorSource"=333, "eRemoteSensorDeviceID"=334, "eSensorTerm"=335, "eRemoteSensorClosedLoopDisableNeutralOnLOS"=336, "ePIDLoopPolarity"=337, "ePIDLoopPeriod"=338, "eSelectedSensorCoefficient"=339, "eForwardSoftLimitThreshold"=340, "eReverseSoftLimitThreshold"=341, "eForwardSoftLimitEnable"=342, "eReverseSoftLimitEnable"=343, "eNominalBatteryVoltage"=350, "eBatterVoltageFilterSize"=351, "eContinuousCurrentLimitAmps"=360, "eContinuousCurrentLimitMs"=361, "ePeakCurrentLimitAmps"=362, "eClosedLoopIAccum"=370, "eCustomParam"=380, "eStickyFaults"=390, "eAnalogPosition"=400, "eQuadraturePosition"=401, "ePulseWidthPosition"=402, "eMotMag_Accel"=410, "eMotMag_VelCruise"=411, "eLimitSwitchSource"=421, "eLimitSwitchNormClosedAndDis"=422, "eLimitSwitchDisabledNeutralOnLOS"=423, "eLimitSwitchRemoteDevID"=424, "eSoftLimitDisabledNeutralOnLOS"=425, "ePulseWidthPeriod_EdgesPerRot"=430, "ePulseWidthPeriod_FilterWindowSz"=431] ("Parameter")
            # "Config Sum 1"
            n28 = call <vilib>:"CTRE_Phoenix_MotorControl_ConfigGetParameter.vi"("timeoutMs"=w135, "ordinal"=1, "Parameter"=w140, "PhoenixMotorControlDevRef"=w137) -> ("error out"=w134:errorcluster, "value"=w138:dbl, "PhoenixMotorControlDevRef"=w132:T12)  [unwired: 5 in]
            n29 = Bundle By Name(cluster=w136, "sum1Term"=w138) -> (w133:T1)
          }
          frame 13 {
            w149 = T17 335 items=["eOnBoot_BrakeMode"=31, "eQuadFilterEn"=91, "eQuadIdxPolarity"=108, "eClearPositionOnIdx"=100, "eMotionProfileHasUnderrunErr"=119, "eMotionProfileTrajectoryPointDurationMs"=120, "eClearPosOnLimitF"=144, "eClearPosOnLimitR"=145, "eStatusFramePeriod"=300, "eOpenLoopRamp"=301, "eClosedLoopRamp"=302, "eNeutralDeadband"=303, "ePeakPosOutput"=305, "eNominalPosOutput"=306, "ePeakNegOutput"=307, "eNominalNegOutput"=308, "eProfileParamSlot_P"=310, "eProfileParamSlot_I"=311, "eProfileParamSlot_D"=312, "eProfileParamSlot_F"=313, "eProfileParamSlot_IZone"=314, "eProfileParamSlot_AllowableErr"=315, "eProfileParamSlot_MaxIAccum"=316, "eProfileParamSlot_PeakOutput"=317, "eClearPositionOnLimitF"=320, "eClearPositionOnLimitR"=321, "eClearPositionOnQuadIdx"=322, "eSampleVelocityPeriod"=325, "eSampleVelocityWindow"=326, "eFeedbackSensorType"=330, "eSelectedSensorPosition"=331, "eFeedbackNotContinuous"=332, "eRemoteSensorSource"=333, "eRemoteSensorDeviceID"=334, "eSensorTerm"=335, "eRemoteSensorClosedLoopDisableNeutralOnLOS"=336, "ePIDLoopPolarity"=337, "ePIDLoopPeriod"=338, "eSelectedSensorCoefficient"=339, "eForwardSoftLimitThreshold"=340, "eReverseSoftLimitThreshold"=341, "eForwardSoftLimitEnable"=342, "eReverseSoftLimitEnable"=343, "eNominalBatteryVoltage"=350, "eBatterVoltageFilterSize"=351, "eContinuousCurrentLimitAmps"=360, "eContinuousCurrentLimitMs"=361, "ePeakCurrentLimitAmps"=362, "eClosedLoopIAccum"=370, "eCustomParam"=380, "eStickyFaults"=390, "eAnalogPosition"=400, "eQuadraturePosition"=401, "ePulseWidthPosition"=402, "eMotMag_Accel"=410, "eMotMag_VelCruise"=411, "eLimitSwitchSource"=421, "eLimitSwitchNormClosedAndDis"=422, "eLimitSwitchDisabledNeutralOnLOS"=423, "eLimitSwitchRemoteDevID"=424, "eSoftLimitDisabledNeutralOnLOS"=425, "ePulseWidthPeriod_EdgesPerRot"=430, "ePulseWidthPeriod_FilterWindowSz"=431] ("Parameter")
            # "Config Diff 0"
            n30 = call <vilib>:"CTRE_Phoenix_MotorControl_ConfigGetParameter.vi"("timeoutMs"=w141, "ordinal"=2, "Parameter"=w149, "PhoenixMotorControlDevRef"=w142) -> ("error out"=w145:errorcluster, "value"=w147:dbl, "PhoenixMotorControlDevRef"=w144:T12)  [unwired: 5 in]
            n31 = Bundle By Name(cluster=w143, "diff0Term"=w147) -> (w146:T1)
          }
          frame 14 {
            w158 = T17 335 items=["eOnBoot_BrakeMode"=31, "eQuadFilterEn"=91, "eQuadIdxPolarity"=108, "eClearPositionOnIdx"=100, "eMotionProfileHasUnderrunErr"=119, "eMotionProfileTrajectoryPointDurationMs"=120, "eClearPosOnLimitF"=144, "eClearPosOnLimitR"=145, "eStatusFramePeriod"=300, "eOpenLoopRamp"=301, "eClosedLoopRamp"=302, "eNeutralDeadband"=303, "ePeakPosOutput"=305, "eNominalPosOutput"=306, "ePeakNegOutput"=307, "eNominalNegOutput"=308, "eProfileParamSlot_P"=310, "eProfileParamSlot_I"=311, "eProfileParamSlot_D"=312, "eProfileParamSlot_F"=313, "eProfileParamSlot_IZone"=314, "eProfileParamSlot_AllowableErr"=315, "eProfileParamSlot_MaxIAccum"=316, "eProfileParamSlot_PeakOutput"=317, "eClearPositionOnLimitF"=320, "eClearPositionOnLimitR"=321, "eClearPositionOnQuadIdx"=322, "eSampleVelocityPeriod"=325, "eSampleVelocityWindow"=326, "eFeedbackSensorType"=330, "eSelectedSensorPosition"=331, "eFeedbackNotContinuous"=332, "eRemoteSensorSource"=333, "eRemoteSensorDeviceID"=334, "eSensorTerm"=335, "eRemoteSensorClosedLoopDisableNeutralOnLOS"=336, "ePIDLoopPolarity"=337, "ePIDLoopPeriod"=338, "eSelectedSensorCoefficient"=339, "eForwardSoftLimitThreshold"=340, "eReverseSoftLimitThreshold"=341, "eForwardSoftLimitEnable"=342, "eReverseSoftLimitEnable"=343, "eNominalBatteryVoltage"=350, "eBatterVoltageFilterSize"=351, "eContinuousCurrentLimitAmps"=360, "eContinuousCurrentLimitMs"=361, "ePeakCurrentLimitAmps"=362, "eClosedLoopIAccum"=370, "eCustomParam"=380, "eStickyFaults"=390, "eAnalogPosition"=400, "eQuadraturePosition"=401, "ePulseWidthPosition"=402, "eMotMag_Accel"=410, "eMotMag_VelCruise"=411, "eLimitSwitchSource"=421, "eLimitSwitchNormClosedAndDis"=422, "eLimitSwitchDisabledNeutralOnLOS"=423, "eLimitSwitchRemoteDevID"=424, "eSoftLimitDisabledNeutralOnLOS"=425, "ePulseWidthPeriod_EdgesPerRot"=430, "ePulseWidthPeriod_FilterWindowSz"=431] ("Parameter")
            # "Config Diff 1"
            n32 = call <vilib>:"CTRE_Phoenix_MotorControl_ConfigGetParameter.vi"("timeoutMs"=w153, "ordinal"=3, "Parameter"=w158, "PhoenixMotorControlDevRef"=w155) -> ("error out"=w151:errorcluster, "value"=w156:dbl, "PhoenixMotorControlDevRef"=w150:T12)  [unwired: 5 in]
            n33 = Bundle By Name(cluster=w154, "diff1Term"=w156) -> (w152:T1)
          }
          frame 15 {
            w167 = T17 362 items=["eOnBoot_BrakeMode"=31, "eQuadFilterEn"=91, "eQuadIdxPolarity"=108, "eClearPositionOnIdx"=100, "eMotionProfileHasUnderrunErr"=119, "eMotionProfileTrajectoryPointDurationMs"=120, "eClearPosOnLimitF"=144, "eClearPosOnLimitR"=145, "eStatusFramePeriod"=300, "eOpenLoopRamp"=301, "eClosedLoopRamp"=302, "eNeutralDeadband"=303, "ePeakPosOutput"=305, "eNominalPosOutput"=306, "ePeakNegOutput"=307, "eNominalNegOutput"=308, "eProfileParamSlot_P"=310, "eProfileParamSlot_I"=311, "eProfileParamSlot_D"=312, "eProfileParamSlot_F"=313, "eProfileParamSlot_IZone"=314, "eProfileParamSlot_AllowableErr"=315, "eProfileParamSlot_MaxIAccum"=316, "eProfileParamSlot_PeakOutput"=317, "eClearPositionOnLimitF"=320, "eClearPositionOnLimitR"=321, "eClearPositionOnQuadIdx"=322, "eSampleVelocityPeriod"=325, "eSampleVelocityWindow"=326, "eFeedbackSensorType"=330, "eSelectedSensorPosition"=331, "eFeedbackNotContinuous"=332, "eRemoteSensorSource"=333, "eRemoteSensorDeviceID"=334, "eSensorTerm"=335, "eRemoteSensorClosedLoopDisableNeutralOnLOS"=336, "ePIDLoopPolarity"=337, "ePIDLoopPeriod"=338, "eSelectedSensorCoefficient"=339, "eForwardSoftLimitThreshold"=340, "eReverseSoftLimitThreshold"=341, "eForwardSoftLimitEnable"=342, "eReverseSoftLimitEnable"=343, "eNominalBatteryVoltage"=350, "eBatterVoltageFilterSize"=351, "eContinuousCurrentLimitAmps"=360, "eContinuousCurrentLimitMs"=361, "ePeakCurrentLimitAmps"=362, "eClosedLoopIAccum"=370, "eCustomParam"=380, "eStickyFaults"=390, "eAnalogPosition"=400, "eQuadraturePosition"=401, "ePulseWidthPosition"=402, "eMotMag_Accel"=410, "eMotMag_VelCruise"=411, "eLimitSwitchSource"=421, "eLimitSwitchNormClosedAndDis"=422, "eLimitSwitchDisabledNeutralOnLOS"=423, "eLimitSwitchRemoteDevID"=424, "eSoftLimitDisabledNeutralOnLOS"=425, "ePulseWidthPeriod_EdgesPerRot"=430, "ePulseWidthPeriod_FilterWindowSz"=431] ("Parameter")
            # "Config Peak Current"
            n34 = call <vilib>:"CTRE_Phoenix_MotorControl_ConfigGetParameter.vi"("timeoutMs"=w162, "ordinal"=0, "Parameter"=w167, "PhoenixMotorControlDevRef"=w164) -> ("error out"=w161:errorcluster, "value"=w165:dbl, "PhoenixMotorControlDevRef"=w159:T12)  [unwired: 5 in]
            n35 = Bundle By Name(cluster=w163, "peakCurrentLimit"=w165) -> (w160:T1)
          }
          frame 16 {
            w176 = T17 361 items=["eOnBoot_BrakeMode"=31, "eQuadFilterEn"=91, "eQuadIdxPolarity"=108, "eClearPositionOnIdx"=100, "eMotionProfileHasUnderrunErr"=119, "eMotionProfileTrajectoryPointDurationMs"=120, "eClearPosOnLimitF"=144, "eClearPosOnLimitR"=145, "eStatusFramePeriod"=300, "eOpenLoopRamp"=301, "eClosedLoopRamp"=302, "eNeutralDeadband"=303, "ePeakPosOutput"=305, "eNominalPosOutput"=306, "ePeakNegOutput"=307, "eNominalNegOutput"=308, "eProfileParamSlot_P"=310, "eProfileParamSlot_I"=311, "eProfileParamSlot_D"=312, "eProfileParamSlot_F"=313, "eProfileParamSlot_IZone"=314, "eProfileParamSlot_AllowableErr"=315, "eProfileParamSlot_MaxIAccum"=316, "eProfileParamSlot_PeakOutput"=317, "eClearPositionOnLimitF"=320, "eClearPositionOnLimitR"=321, "eClearPositionOnQuadIdx"=322, "eSampleVelocityPeriod"=325, "eSampleVelocityWindow"=326, "eFeedbackSensorType"=330, "eSelectedSensorPosition"=331, "eFeedbackNotContinuous"=332, "eRemoteSensorSource"=333, "eRemoteSensorDeviceID"=334, "eSensorTerm"=335, "eRemoteSensorClosedLoopDisableNeutralOnLOS"=336, "ePIDLoopPolarity"=337, "ePIDLoopPeriod"=338, "eSelectedSensorCoefficient"=339, "eForwardSoftLimitThreshold"=340, "eReverseSoftLimitThreshold"=341, "eForwardSoftLimitEnable"=342, "eReverseSoftLimitEnable"=343, "eNominalBatteryVoltage"=350, "eBatterVoltageFilterSize"=351, "eContinuousCurrentLimitAmps"=360, "eContinuousCurrentLimitMs"=361, "ePeakCurrentLimitAmps"=362, "eClosedLoopIAccum"=370, "eCustomParam"=380, "eStickyFaults"=390, "eAnalogPosition"=400, "eQuadraturePosition"=401, "ePulseWidthPosition"=402, "eMotMag_Accel"=410, "eMotMag_VelCruise"=411, "eLimitSwitchSource"=421, "eLimitSwitchNormClosedAndDis"=422, "eLimitSwitchDisabledNeutralOnLOS"=423, "eLimitSwitchRemoteDevID"=424, "eSoftLimitDisabledNeutralOnLOS"=425, "ePulseWidthPeriod_EdgesPerRot"=430, "ePulseWidthPeriod_FilterWindowSz"=431] ("Parameter")
            # "Config Peak Current"
            n36 = call <vilib>:"CTRE_Phoenix_MotorControl_ConfigGetParameter.vi"("timeoutMs"=w171, "ordinal"=0, "Parameter"=w176, "PhoenixMotorControlDevRef"=w173) -> ("error out"=w170:errorcluster, "value"=w174:dbl, "PhoenixMotorControlDevRef"=w168:T12)  [unwired: 5 in]
            n37 = Bundle By Name(cluster=w172, "peakCurrentDuration"=w174) -> (w169:T1)
          }
          frame 17 {
            w185 = T17 360 items=["eOnBoot_BrakeMode"=31, "eQuadFilterEn"=91, "eQuadIdxPolarity"=108, "eClearPositionOnIdx"=100, "eMotionProfileHasUnderrunErr"=119, "eMotionProfileTrajectoryPointDurationMs"=120, "eClearPosOnLimitF"=144, "eClearPosOnLimitR"=145, "eStatusFramePeriod"=300, "eOpenLoopRamp"=301, "eClosedLoopRamp"=302, "eNeutralDeadband"=303, "ePeakPosOutput"=305, "eNominalPosOutput"=306, "ePeakNegOutput"=307, "eNominalNegOutput"=308, "eProfileParamSlot_P"=310, "eProfileParamSlot_I"=311, "eProfileParamSlot_D"=312, "eProfileParamSlot_F"=313, "eProfileParamSlot_IZone"=314, "eProfileParamSlot_AllowableErr"=315, "eProfileParamSlot_MaxIAccum"=316, "eProfileParamSlot_PeakOutput"=317, "eClearPositionOnLimitF"=320, "eClearPositionOnLimitR"=321, "eClearPositionOnQuadIdx"=322, "eSampleVelocityPeriod"=325, "eSampleVelocityWindow"=326, "eFeedbackSensorType"=330, "eSelectedSensorPosition"=331, "eFeedbackNotContinuous"=332, "eRemoteSensorSource"=333, "eRemoteSensorDeviceID"=334, "eSensorTerm"=335, "eRemoteSensorClosedLoopDisableNeutralOnLOS"=336, "ePIDLoopPolarity"=337, "ePIDLoopPeriod"=338, "eSelectedSensorCoefficient"=339, "eForwardSoftLimitThreshold"=340, "eReverseSoftLimitThreshold"=341, "eForwardSoftLimitEnable"=342, "eReverseSoftLimitEnable"=343, "eNominalBatteryVoltage"=350, "eBatterVoltageFilterSize"=351, "eContinuousCurrentLimitAmps"=360, "eContinuousCurrentLimitMs"=361, "ePeakCurrentLimitAmps"=362, "eClosedLoopIAccum"=370, "eCustomParam"=380, "eStickyFaults"=390, "eAnalogPosition"=400, "eQuadraturePosition"=401, "ePulseWidthPosition"=402, "eMotMag_Accel"=410, "eMotMag_VelCruise"=411, "eLimitSwitchSource"=421, "eLimitSwitchNormClosedAndDis"=422, "eLimitSwitchDisabledNeutralOnLOS"=423, "eLimitSwitchRemoteDevID"=424, "eSoftLimitDisabledNeutralOnLOS"=425, "ePulseWidthPeriod_EdgesPerRot"=430, "ePulseWidthPeriod_FilterWindowSz"=431] ("Parameter")
            n38 = call <vilib>:"CTRE_Phoenix_MotorControl_ConfigGetParameter.vi"("timeoutMs"=w180, "ordinal"=0, "Parameter"=w185, "PhoenixMotorControlDevRef"=w182) -> ("error out"=w179:errorcluster, "value"=w183:dbl, "PhoenixMotorControlDevRef"=w177:T12)  [unwired: 5 in]
            n39 = Bundle By Name(cluster=w181, "continuousCurrentLimit"=w183) -> (w178:T1)
          }
          frame Default {
          }
        }
      }
      n40 = Or Array Elements(Boolean array=w11) -> (logical OR=w14:bool)
      n41 = Select(t=errorcluster {"status"=TRUE, "code"=-1, "source"="Motor Controller Get Configs Enhanced: 1 or more configs failed"} ("error out 2"), s=w14, f=errorcluster {"status"=FALSE, "code"=0, "source"=""} ("error out 2")) -> (s? t:f=w15:errorcluster)
    }
    frame Error {
    }
  }
  "PhoenixMotorControlDevRef" <- w5
  "error out" <- w7
  "Enhanced Motor Controller Configurables" <- w2
